vi "AK Befehl Auswerten_v1.4.vi"(10 "Array":string[](array[string])) -> (2 "String für schreiben":string)   [LabVIEW 2020, in "AK-Schnittstelle.lvlib"]
uses:
  AK-Schnittstelle.lvlib
  Aktionen Stoernummern pruefen.ctl
  Aktionen Zustandsfehlerinformation.ctl
  Aktionen Gespeicherte Werte.ctl
  Seiten/Anlagengrenzwerte/FGV Anlagengrenzwerte Aktionen.ctl
  Seiten/FT-IR/FGV FT-IR Diagnose Aktionen.ctl
  Funktionstasten/Funktionstasten-Aktion.ctl
  Seiten/System Einstellungen V2/Aktioen FGV System Konstanten.ctl
  AK Namen Aktionen.ctl
  Seiten/System Einstellungen V2/Aktioen FGV System.ctl
  Funktionstasten/Zustaende.ctl
  Seiten/Erweiterte Konfig/Status Dichtheitstest Aktionen.ctl
  Seiten/Erweiterte Konfig/FGV PID Aktionen.ctl
  Seiten/FT-IR/FGV FT-IR Aktionen.ctl
  Seiten/FT-IR/Aktion FGV Rezepte wechseln.ctl
  Seiten/FT-IR/FGV FT-IR Gasliste Aktionen.ctl
  Seiten/FT-IR/Span/Aktion FGV SGSF und SGSO weiterleiten.ctl
  Seiten/FT-IR/AK interface/Kommandos verwalten Aktionen.ctl
  Schedule Modul/Aktion FGV Scheduler Status.ctl
  PNS/Aktionen FGV Istwerte.ctl
  Funktionstasten/Betriebsart.ctl
  Seiten/FT-IR/Span/Aktion FGV Span.ctl
  Messdaten/Aktionen FGV Messdaten.ctl
  Seiten/FT-IR/AK-manuell.ctl
  Aktion FGV Spektren automatisch aufzeichnen.ctl
  Seiten/Log Konfig/Aktionen Trigger.ctl
  Seiten/Erweiterte Konfig/Dichtheitstest.vi
  Seiten/FT-IR/TOOLweb Interface Library/TOOLweb Rezept wechseln.vi
  Funktionstasten/Funktionstasten.lvlib
  Seiten/Log Konfig/LogKonfig.lvlib
  Seiten/FT-IR/FT-IR.lvlib
  Messdaten/Messdaten.lvlib
  Seiten/System Einstellungen V2/System Einstellungen V2.lvlib
  Seiten/Erweiterte Konfig/Erweiterte Konfig.lvlib
  Allgemein/allgemeine Sub-VIs.lvlib
  cRIO/PC/Kommunikation mit cRIO.lvlib
  Seiten/Anlagengrenzwerte/Anlagengrenzwerte.lvlib
  Seiten/FT-IR/TOOLweb Interface Library/TOOLweb Interface.lvlib
  PNS/PNS.lvlib
  Schedule Modul/Schedule Modul.lvlib
  Seiten/FT-IR/Span/Spanfaktor.lvlib
  Seiten/FT-IR/AK interface/AK-Interface.lvlib
  EPA 1065/Dichtheitstest 1065-345/Aktion Protokolldaten_Leak check.ctl
  EPA 1065/Dichtheitstest 1065-345/Dichtheitstest 1065-345.lvlib
  EPA 1065/Dichtheitstest 1065-345/Aktion FGV Automatic start.ctl
  Bildwechsel/Bild-Auswahl.ctl
  Bildwechsel/Bildwechsel.lvlib
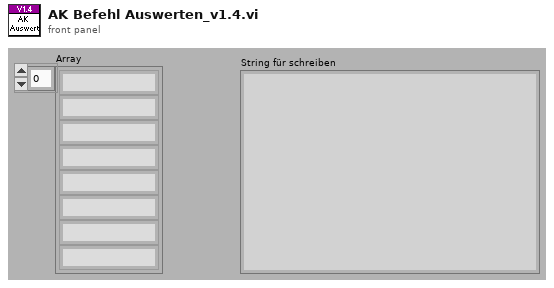
[diagram p1: front panel]
types:
  T1 = typedef "AK-Schnittstelle.lvlib/Aktionen Stoernummern pruefen.ctl" = enum16{"lesen", "prüfen"}
  T2 = typedef "AK-Schnittstelle.lvlib/Aktionen Zustandsfehlerinformation.ctl" = enum16{"OK", "Offline", "Busy", "Syntax Error", "Datenfehler"}
  T3 = typedef "AK-Schnittstelle.lvlib/Aktionen Gespeicherte Werte.ctl" = enum16{"lesen", "laden", "speichern", "Seriell", "TCP", "Diverse", "AKTIV", "AK-Namen"}
  T4 = typedef "Anlagengrenzwerte.lvlib/FGV Anlagengrenzwerte Aktionen.ctl" = enum16{"Lesen", "Grenzwerte schreiben"}
  T5 = typedef "FT-IR.lvlib/FGV FT-IR Diagnose Aktionen.ctl" = enum16{"Lesen", "Diagnose Schreiben", "Min Schreiben", "Max Schreiben"}
  T6 = typedef "Funktionstasten.lvlib/Funktionstasten-Aktion.ctl" = enum16{"Initialisieren", "Zustand setzen", "Taste gedrückt", "Fehler speichern", "Lesen", "Manuell", "Remote", "Bitparallel", "Samplepoint", "Zeit Prüfen", "reset Umschalten"}
  T7 = typedef "System Einstellungen V2.lvlib/Aktioen FGV System Konstanten.ctl" = enum16{"lesen", "laden", "speichern", "Sprache"}
  T8 = typedef "AK-Schnittstelle.lvlib/AK Namen Aktionen.ctl" = enum16{"lesen", "laden", "speichern Namen", "AK Namen", "Liste erstellen", "EKFG erstellen", "speichern EKFG", "EKFG schreiben", "Neuen Eintrag erzeugen"}
  T9 = typedef "FT-IR.lvlib/FGV FT-IR Gasliste Aktionen.ctl" = enum16{"lesen", "Gasliste FT-IR", "Gasliste ausgelesen", "laden", "speichern", "löschen"}
  T10 = typedef "System Einstellungen V2.lvlib/Aktioen FGV System.ctl" = enum16{"lesen", "laden", "speichern", "Optionen schreiben", "Zeitstempel", "Reset BMP", "Reset SQP", "Wartung", "Werkseinstellung"}
  T11 = typedef "Messdaten.lvlib/Aktionen FGV Messdaten.ctl" = enum16{"lesen", "schreiben", "löschen", "Mittelwerte", "Komponente"}
  T12 = typedef "Funktionstasten.lvlib/Zustaende.ctl" = enum16{"Standby", "Pause", "Eco", "Messen", "Kalibrieren", "Spülen Filter", "Spülen Leitung", "Umgebungsluft", "0-Gas", "Cal-Gas", "CG zu PNS", "-------------", "Init 1", "Init 2", "Init 3", "Init 4", "Messen vorbereiten", "Messen durchführen", "Exit"}
  T13 = typedef "EPA 1065.lvlib/Dichtheitstest 1065-345.lvlib/Aktion Protokolldaten_Leak check.ctl" = enum16{"lesen", "Zeitstempel", "Bearbeiter", "Daten", "Auswertung", "löschen"}
  T14 = typedef "Erweiterte Konfig.lvlib/Status Dichtheitstest Aktionen.ctl" = enum16{"lesen", "Zeitstempel", "Daten", "läuft", "Protokolldaten"}
  T15 = typedef "Erweiterte Konfig.lvlib/FGV PID Aktionen.ctl" = enum16{"Lesen", "Schreiben PID", "Schreiben Sonstige", "Dichtheitstest", "Aktionen Dicht.", "Parameter Sensor"}
  T16 = typedef "FT-IR.lvlib/FGV FT-IR Aktionen.ctl" = enum16{"lesen", "NOG setzen", "NOS setzen", "Initialisieren", "speichern", "ALLES setzen", "FT-IR Spektrum loggen", "Komm Stoppen", "Spektrum LogKonfig"}
  T17 = typedef "FT-IR.lvlib/Aktion FGV Rezepte wechseln.ctl" = enum16{"lesen", "Rezepte", "Rezeptindex", "Diesel", "Gasoline", "NCG", "laden", "speichern", "AK/Man"}
  T18 = typedef "FT-IR.lvlib/Spanfaktor.lvlib/Aktion FGV SGSF und SGSO weiterleiten.ctl" = enum16{"lesen", "AGSF", "AGSO", "AGSF löschen", "AGSO löschen", "SGSF", "SGSO", "SGSF löschen", "SGSO löschen"}
  T19 = typedef "FT-IR.lvlib/AK-Interface.lvlib/Kommandos verwalten Aktionen.ctl" = enum16{"lesen", "setzen Ende", "setzen Pos1", "senden", "initalisieren", "prüfen", "Kommandos"}
  T20 = typedef "Schedule Modul.lvlib/Aktion FGV Scheduler Status.ctl" = enum16{"lesen", "init", "aktiv", "inaktiv"}
  T21 = typedef "PNS.lvlib/Aktionen FGV Istwerte.ctl" = enum16{"lesen", "initialisieren", "schreiben", "Störungen"}
  T22 = typedef "Funktionstasten.lvlib/Betriebsart.ctl" = enum16{"Manuell", "Remote", "Bitparallel"}
  T23 = typedef "FT-IR.lvlib/Spanfaktor.lvlib/Aktion FGV Span.ctl" = enum16{"lesen", "Span", "Seite aktiv", "Offset", "FGV aktualisiert", "Aktualisierung aufheben"}
  T24 = typedef "EPA 1065.lvlib/Dichtheitstest 1065-345.lvlib/Aktion FGV Automatic start.ctl" = enum16{"lesen", "Test starten aktiv", "Test starten inaktiv", "Seite merken", "Seite zurücksetzen", "AK Start inaktiv"}
  T25 = typedef "Bildwechsel.lvlib/Bild-Auswahl.ctl" = enum16{"lesen", "Initialisieren", "Beenden", "Grafik", "Anlagenübersicht", "Anlagengrenzwerte", "Log Konfig", "Gaszuordnung AO", "Erw. Konfiguration", "FT-IR  ", "Störmeldungen", "Störmeldepuffer", "Störmeldekonfig", "PNS Grenzwerte", "Statusübersicht", "Linearisierung", "ARN", "EPA Dichtheitstest", "FID", "PMA", "CalGas", "Lambda", "Interference", "Amium PNS", "EPA T90", "Interference N2O", "Scheduler", "Systemeinstellungen", "EPA Drift"}
  T26 = typedef "FT-IR.lvlib/AK-manuell.ctl" = enum16{"manuell", "Diesel", "CNG", "Gasoline"}
  T27 = typedef "AK-Schnittstelle.lvlib/Aktion FGV Spektren automatisch aufzeichnen.ctl" = enum16{"init", "lesen", "prüfen", "set", "reset"}
  T28 = typedef "LogKonfig.lvlib/Aktionen Trigger.ctl" = enum16{"lesen", "ALLE schreiben", "Trigger prüfen", "Trigger rücksetzen"}
  T29 = typedef "AK-Schnittstelle.lvlib/Diverse gespeicherte Werte.ctl" = cluster{"Kalibriergaseingang":i16, "SamplePoint":i16, "CalGas zu PNS":i16, "Gas-Reihenfolge":i16[], "Zeit 0-Gas":sgl, "Zeit CalGas":sgl, "AK Befehlssatz":T30}
  T30 = typedef "AK-Schnittstelle.lvlib/AK Befehlssatz.ctl" = enum16{"MEXA", "IAG v1.4", "AVL (Puma)", "PEUS"}
  T31 = typedef "Anlagengrenzwerte.lvlib/Anlagen-Grenzwerte Anzeige.ctl" = cluster{"Eingangsdruck FT-IR:":T32, "Durchfluss FT-IR:":T32, "Durchfluss CalGas:":T32, "Druck Ausgang:":T32, "Druck Kalter Block:":T32, "Heizleitungen intern:":T32, "Heizleitung zu FT-IR:":T32, "Heizung Filterblock:":T32, "Heizung Pumpe:":T32, "Heizleitung Extern SP1:":T32, "Heizleitung Extern SP2:":T32, "FT-IR Heizung Messzelle:":T32, "Schaltschranktemperatur:":T32, "Gaskühler:":T32}
  T32 = typedef "Anlagengrenzwerte.lvlib/Anlagen-Parameter Anzeige.ctl" = cluster{"Sollwert":sgl, "Warn-Min":sgl, "Warn-Max":sgl, "Abschalt-Min":sgl, "Abschalt-Max":sgl, "Regler":u16}
  T33 = typedef "Verwaltung - cRIO.lvlib/Analog Eingaenge.ctl" = cluster{"AI0: Durchfluss FT-IR":sgl, "AI1: Druck Ausgang":sgl, "AI2: Umgebungsdruck":sgl, "AI3: Druck FT-IR":sgl, "AI4: Druck CalGas":sgl, "AI5: Reserve":sgl, "AI6: Reserve":sgl, "AI7: Reserve":sgl, "Rohwert Durchfluss FT-IR":sgl, "Rohwert Druck Ausgang":sgl, "Rohwert Umgebungsdruck":sgl, "Rohwert Druck FT-IR":sgl, "Rohwert Druck CalGas":sgl, "Rohwert AI5":sgl, "Rohwert AI6":sgl, "Rohwert AI7":sgl, "Rohwert Diffdruck mbar FTIR":sgl}
  T34 = typedef "FT-IR.lvlib/TOOLweb Interface.lvlib/Typdefinitionen.lvlib/TOOLweb Diagnose.ctl" = cluster{"(14) temperature":sgl, "(15) pressure":sgl, "(16) oxygen":sgl, "(50) diag-igramdc":sgl, "(51) diag-igrampp":sgl, "(52) diag-phaseAngle":sgl, "(53) diag-laserpp":sgl, "(54) diag-laserdc":sgl, "(55) diag-badscan":sgl, "(56) diag-centerburst":sgl, "(57) diag-linearizerCheck":sgl, "(58) diag-SNR":sgl, "(59) diag-sBeamIntensity":sgl}
  T35 = cluster{"Modell":string, "ProjektNummer":string, "Software Version":string, "Seriennummer":string}
  T36 = typedef "String - Ausgabefeld.ctl" = string
  T37 = typedef "System Einstellungen V2.lvlib/Optionen.ctl" = cluster{"Störmeldep.":bool, "Betriebszustände":bool, "AK in ppm":bool, "log Cal-Gas":bool, "log 0-Gas":bool, "Durchflusssensor 0-5V":bool, "PNS?":bool, "Mit N2 spülen":bool, "TRE08":bool, "Amium 10-Fach":bool, "Verticale Scrollbar aktiv":bool, "Loggingtakt":bool, "AK Rezeptwechsel gleich wie MKS":bool, "NG ECO":bool}
  T38 = typedef "EPA 1065.lvlib/Dichtheitstest 1065-345.lvlib/Leak Daten.ctl" = cluster{"Gesamtes Volumen":sgl, "p 1":sgl, "p 2":sgl, "T 1":sgl, "T 2":sgl, "t 1":timestamp, "t 2":timestamp, "Ergebnis mol/s":sgl, "Grenze mol/s":sgl, "Leak in %":sgl, "Ergebnis mbar":sgl, "Grenze mbar":sgl}
  T39 = typedef "Erweiterte Konfig.lvlib/Sonstige Parameter.ctl" = cluster{"Lüfter langsam":sgl, "Lüfter schnell":sgl, "FT-IR Kühlung Soll":sgl, "FT-IR Kühlung Max":sgl, "Überwachung":T40, "Befüllung aktiv":T41, "Stickstoff Befüllzeit":sgl, "Befüllintervall":sgl, "Kalibrierwert FT-IR":sgl, "Offset Ausgang":sgl, "Offset FT-IR":sgl, "Offset Druck FT-IR":sgl, "Dichtheitstest Zeit":sgl, "Dichtheitstest Abfall":sgl, "Dichtheitstest Umfang":T42, "Offset Umgebung":sgl, "Max Taupunkt":sgl, "Pumpendrehzahl":sgl, "ext. Befüllung":T41, "Ext. Stickstoff Befüllzeit":sgl}
  T40 = typedef "Auswahlfeld.ctl" = u16
  T41 = typedef "LogKonfig.lvlib/Auswahlfeld aktiviert-deaktiviert.ctl" = u16
  T42 = typedef "Erweiterte Konfig.lvlib/Dichtheitstest Umfang.ctl" = u16
  T43 = cluster{"(80) labEnabled":bool, "(81) labPath":path, "(82) labBaseName":string, "(83) labIndex":string, "Spektrum loggen aktiv?":bool}
  T44 = typedef "Verwaltung - cRIO.lvlib/TC Eingaenge.ctl" = cluster{"TC0: Reserve":sgl, "TC1: HL zu FT-IR":sgl, "TC2: HL Extern SP1":sgl, "TC3: HL Extern SP2":sgl, "TC4: Reserve":sgl, "TC5: Reserve":sgl, "TC6: Reserve":sgl, "TC7: Reserve":sgl, "TC8: FT-IR":sgl, "TC9: Reserve":sgl, "TC10: Schaltschrank":sgl, "TC11: Umgebung":sgl}
  T45 = typedef "Steuerung PNS.lvclass/Regler.ctl" = cluster{"Istwert":i16, "Sollwert":i16, "Alarm MIN":i16, "Alarm MAX":i16, "Regler sperren":i16, "Analog Ausgang":i16}[]
  T46 = cluster{"Istwert":i16, "Sollwert":i16, "Alarm MIN":i16, "Alarm MAX":i16, "Regler sperren":i16, "Analog Ausgang":i16}
  T47 = typedef "LogKonfig.lvlib/Element Triggerereignisse.ctl" = cluster{"Trigger verwenden":T41, "Messwert":u16, "kl./gr.":u16, "Wert":sgl, "Puffergröße":sgl}
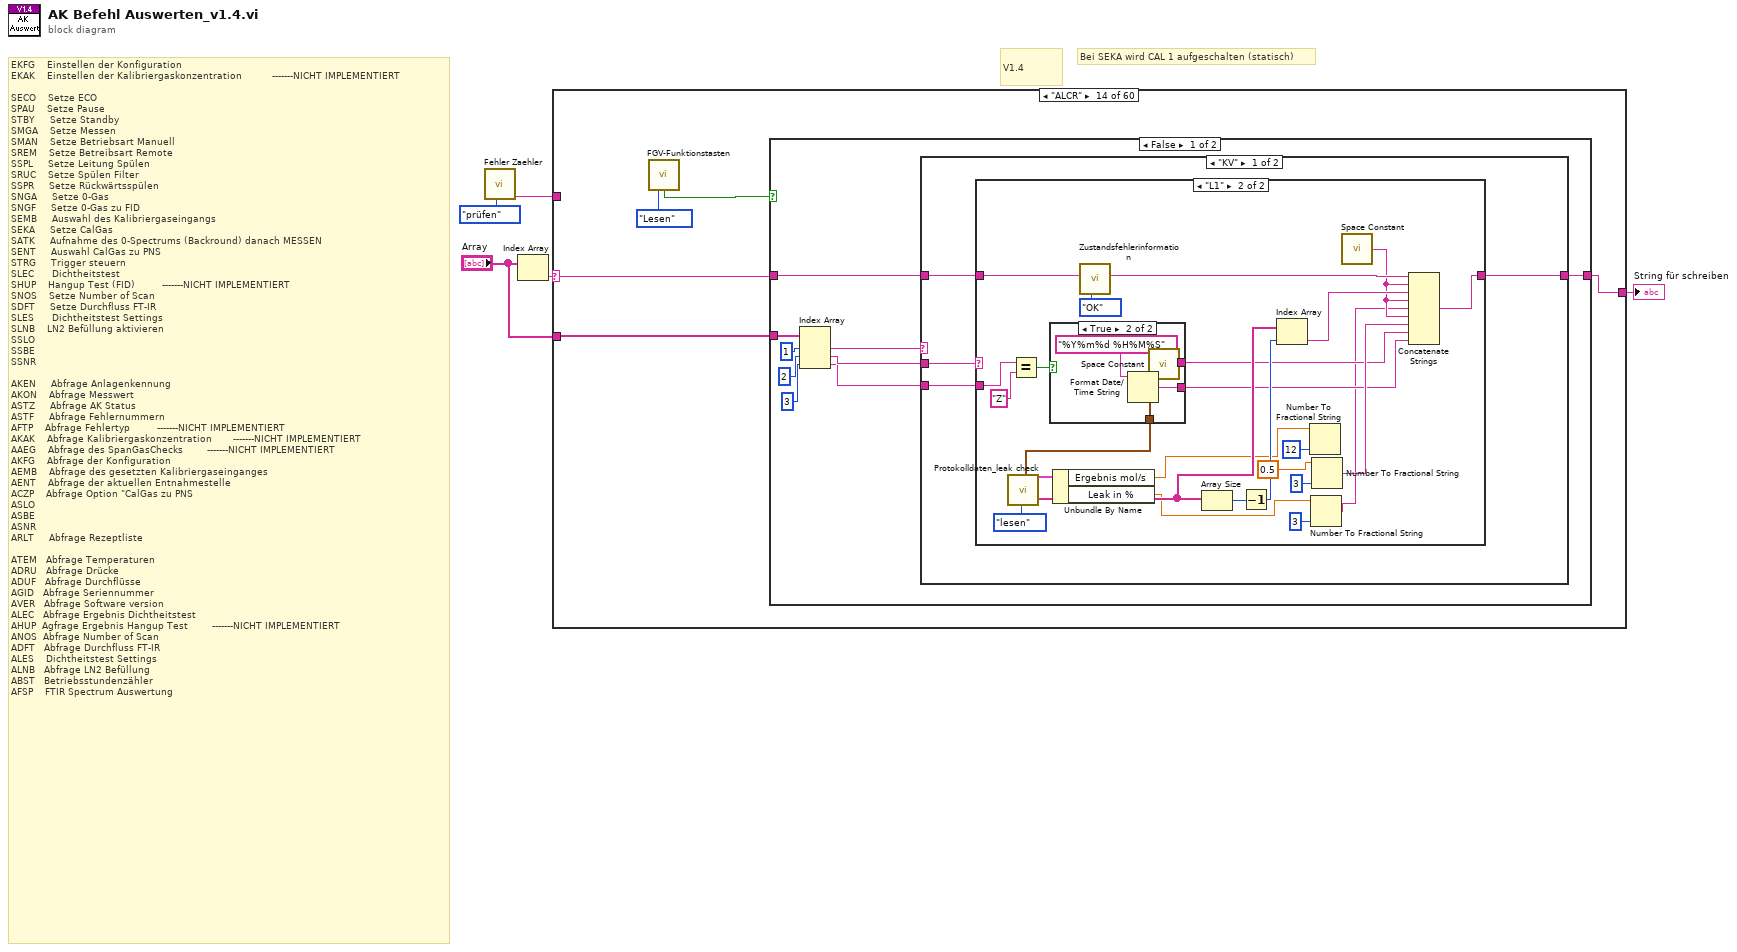
[diagram p0: block diagram]
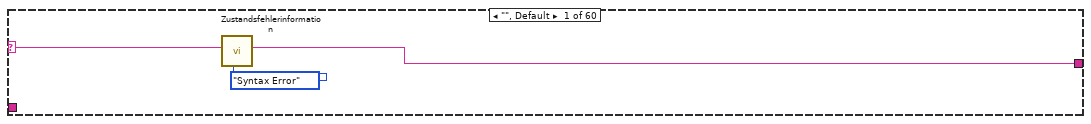
[diagram p2: hidden frame]
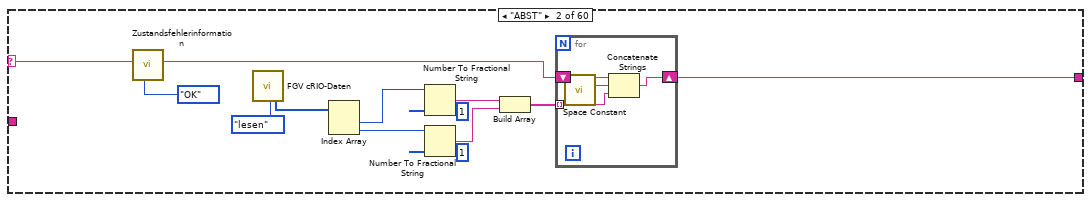
[diagram p3: hidden frame]
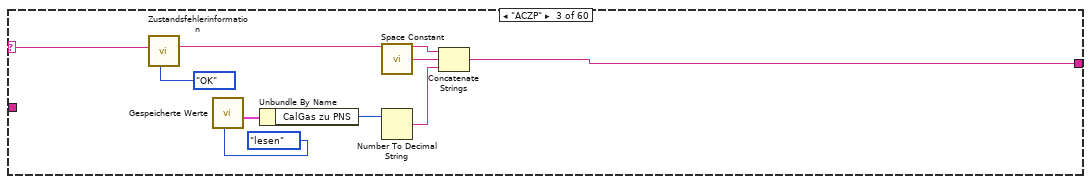
[diagram p4: hidden frame]
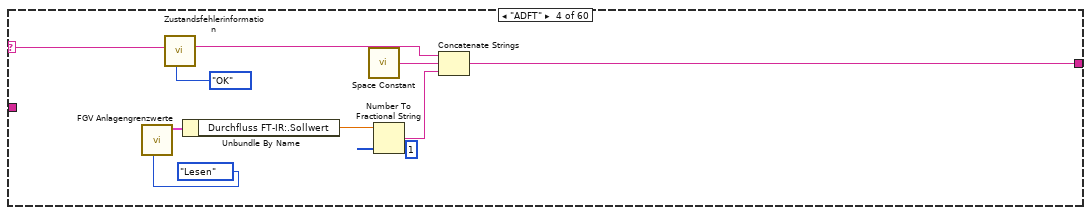
[diagram p5: hidden frame]
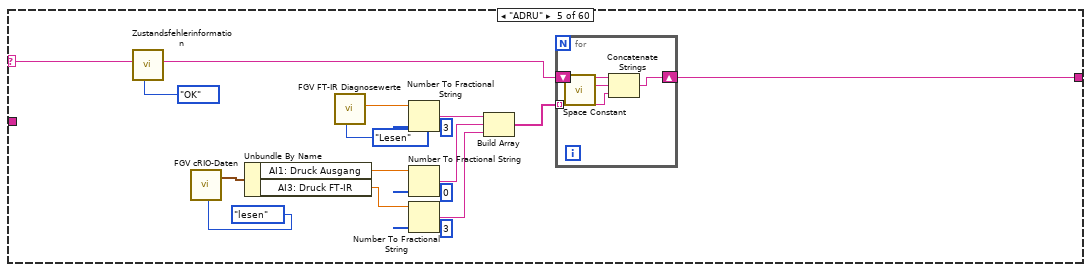
[diagram p6: hidden frame]
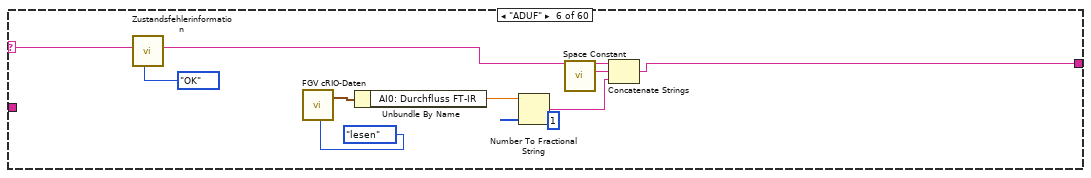
[diagram p7: hidden frame]
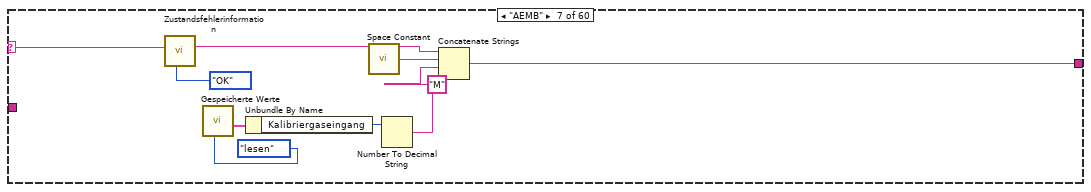
[diagram p8: hidden frame]
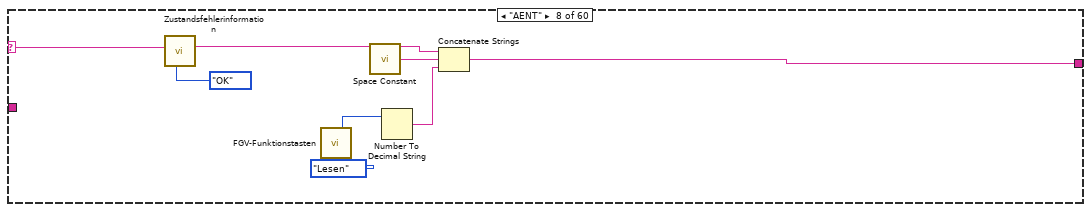
[diagram p9: hidden frame]
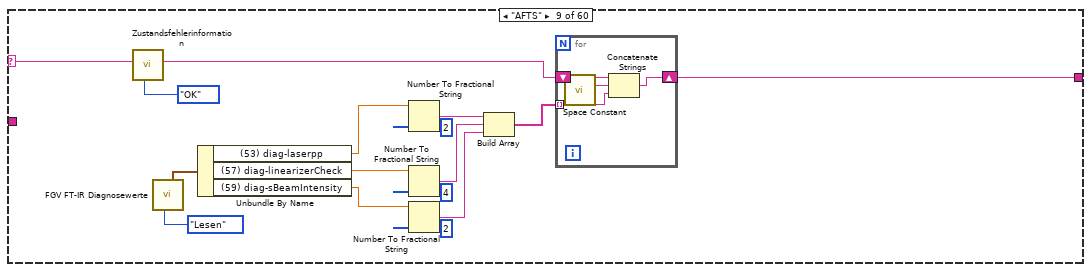
[diagram p10: hidden frame]
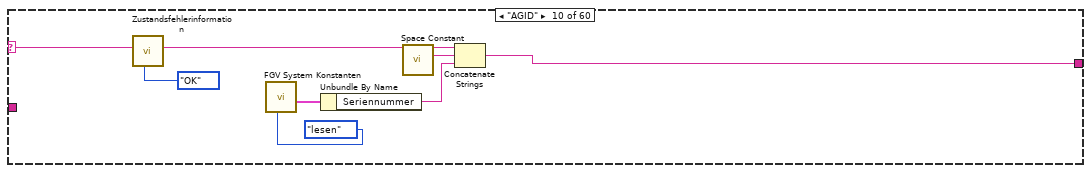
[diagram p11: hidden frame]
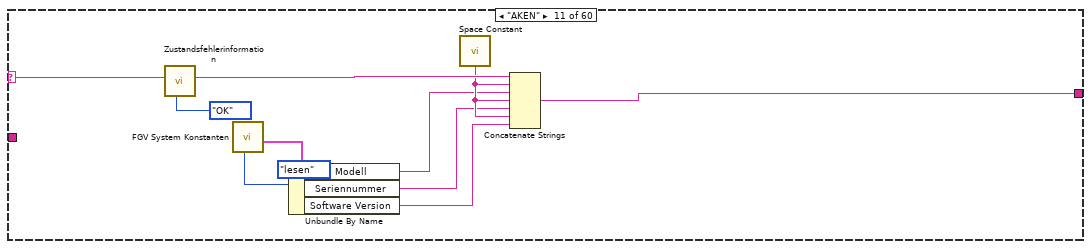
[diagram p12: hidden frame]
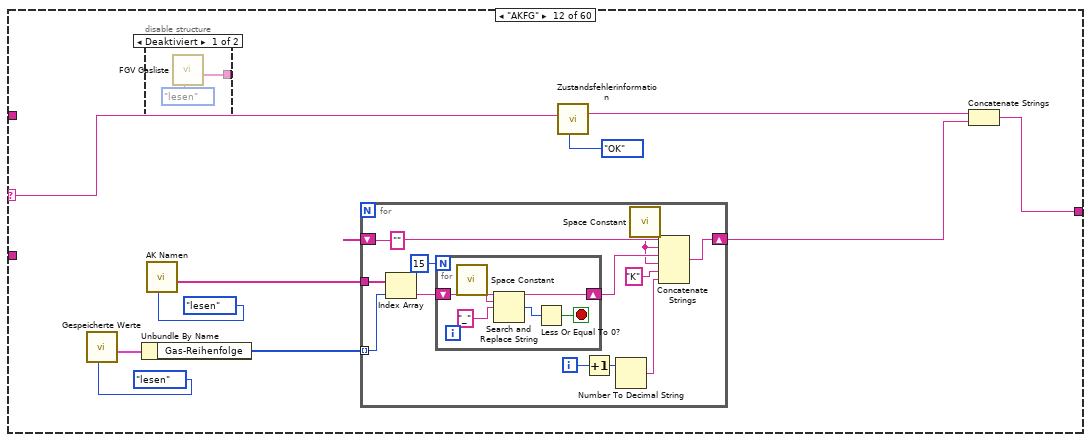
[diagram p13: hidden frame]
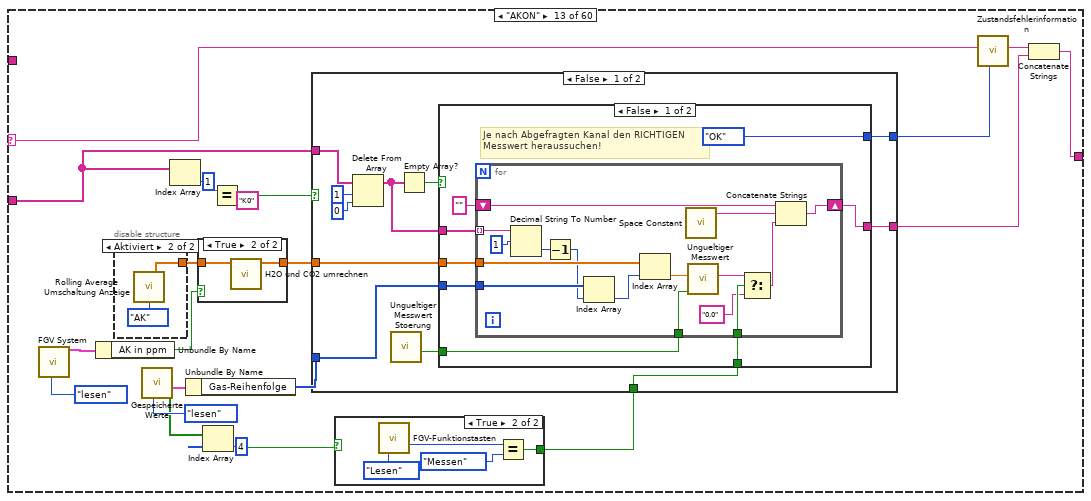
[diagram p15: hidden frame]
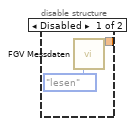
[diagram p16: hidden frame]
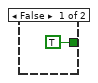
[diagram p17: hidden frame]
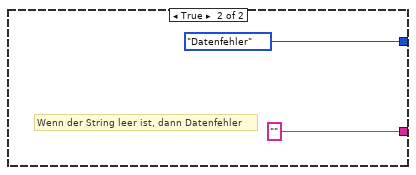
[diagram p19: hidden frame]
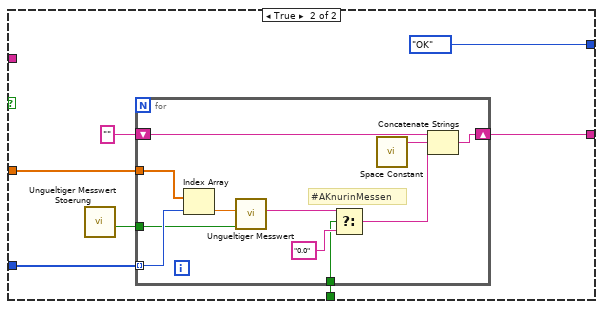
[diagram p20: hidden frame]
diagram:
  # "Bei SEKA wird CAL 1 aufgeschalten (statisch)"
  # "V1.4"
  # "EKFG    Einstellen der Konfiguration\nEKAK    Einstellen der Kalibriergaskonzentration          -------NICHT IMPLEMENTIERT\n\nSECO    Setze ECO\nSPAU    Setze Pause\nSTBY     Setze Standby\nSMGA    Setze Messen\nSMAN    Setze Betriebsart Manuell\nSREM    Setze Betreibsart Remote\nSSPL     Setze Leitung Spülen\nSRUC    Setze Spülen Filter\nSSPR     Setze Rückwärtsspülen\nSNGA     Setze 0-Gas\nSNGF     Setze 0-Gas zu FID\nSEMB     Auswahl des Kalibriergaseingangs\nSEKA     Setze CalGas\nSATK     Aufnahme des 0-Spectrums (Backround) danach MESSEN\nSENT     Auswahl CalGas zu PNS\nSTRG     Trigger steuern\nSLEC      Dichtheitstest\nSHUP    Hangup Test (FID)         -------NICHT IMPLEMENTIERT\nSNOS    Setze Number of Scan\nSDFT     Setze Durchfluss FT-IR\nSLES      Dichtheitstest Settings\nSLNB    LN2 Befüllung aktivieren\nSSLO\nSSBE\nSSNR\n\nAKEN     Abfrage Anlagenkennung\nAKON    Abfrage Messwert\nASTZ     Abfrage AK Status\nASTF     Abfrage Fehlernummern\nAFTP    Abfrage Fehlertyp         -------NICHT IMPLEMENTIERT\nAKAK    Abfrage Kalibriergaskonzentration       -------NICHT IMPLEMENTIERT\nAAEG    Abfrage des SpanGasChecks        -------NICHT IMPLEMENTIERT\nAKFG    Abfrage der Konfiguration\nAEMB    Abfrage des gesetzten Kalibriergaseinganges\nAENT    Abfrage der aktuellen Entnahmestelle\nACZP    Abfrage Option \"CalGas zu PNS\nASLO\nASBE\nASNR\nARLT     Abfrage Rezeptliste\n\nATEM   Abfrage Temperaturen\nADRU   Abfrage Drücke\nADUF   Abfrage Durchflüsse\nAGID   Abfrage Seriennummer\nAVER   Abfrage Software version\nALEC   Abfrage Ergebnis Dichtheitstest\nAHUP  Agfrage Ergebnis Hangup Test        -------NICHT IMPLEMENTIERT\nANOS  Abfrage Number of Scan\nADFT   Abfrage Durchfluss FT-IR\nALES    Dichtheitstest Settings\nALNB   Abfrage LN2 Befüllung\nABST   Betriebsstundenzähler\nAFSP    FTIR Spectrum Auswertung"
  n1 = call "Fehler Zaehler.vi"("Aktionen"=Aktionen_Stoernummern_pruefen."prüfen") -> ("Fehlerzähler"=w3:string)  [unwired: 7 in, 3 out]
  n2 = Index Array(array="Array") -> (element=w2:string)  [unwired: 1 in]
  n3 = case shown="\"ALCR\"" w2 {
    selector: w2 -> [w7 w20 w32 w42 w60 w74 w83 w91 w108 w120 w129 w140 w183 w252 w321 w342 w354 w362 w369 w386 w410 w420 w453 w486 w519 w548 w558 w566 w573 w585 w627 w642 w650 w668 w673 w701 w858 w860 w891 w913 w933 w970 w994 w1045 w1075 w1089 w1099 w1103 w1106 w1137 w1144 w1216 w1228 w1235 w1270 w1320 w1352 w1356 w1359 w1362]
    tunnel: [w6 w18 w34 w44 w55 w71 w85 w93 w106 w116 w131 w142 w184 w253 w314 w340 w356 w364 w371 w373 w399 w416 w449 w482 w515 w550 w560 w568 w575 w587 w620 w638 w649 w667 w672 w700 w857 w859 w890 w912 w934 w969 w993 w1044 w1074 w1088 w1098 w1102 w1105 w1136 w1143 w1215 w1227 w1234 w1269 w1319 w1351 w1355 w1358 w1361] -> w5
    tunnel: w3 -> [_ _ _ _ _ _ _ _ _ _ _ _ _ _ _ _ _ _ _ _ _ _ _ _ _ _ _ _ _ _ _ _ _ _ _ _ _ _ _ _ _ _ _ _ _ _ _ _ _ _ _ _ _ _ _ _ _ _ _ _]
    tunnel: "Array" -> [_ _ _ _ _ _ _ _ _ _ _ _ w174 w254 _ _ _ _ _ _ _ w425 w458 w491 w524 _ _ _ _ _ _ _ w651 _ w671 w705 _ _ w889 w911 w935 _ w992 w1043 _ _ w1097 _ w1104 _ w1145 _ w1220 w1230 w1265 w1315 w1344 _ _ w1360]
    frame "", Default {
      n4 = call "Zustandsfehlerinformation.vi"("Aktionen"=Aktionen_Zustandsfehlerinformation."Syntax Error", "String"=w7) -> ("String"=w6:string)  [unwired: 9 in]
    }
    frame "ABST" {
      n5 = call "Zustandsfehlerinformation.vi"("Aktionen"=Aktionen_Zustandsfehlerinformation."OK", "String"=w20) -> ("String"=w17:string)  [unwired: 9 in]
      n6 = call "FGV cRIO-Daten.vi"("Aktion"=enum16{"lesen", "schreiben"}."lesen") -> ("PID Stellwerte"=w9:i16[])  [unwired: 9 in, 9 out]
      n7 = Index Array(array=w9) -> (element #1=w10:i16, element #2=w11:i16)  [unwired: 2 in]
      n8 = Number To Fractional String(number=w10, precision (6)=i16 1 ("Genauigkeit (6)")) -> (F-format string=w14:string)  [unwired: 2 in]
      n9 = Number To Fractional String(number=w11, precision (6)=i16 1 ("Genauigkeit (6)")) -> (F-format string=w13:string)  [unwired: 2 in]
      n10 = Build Array(w14, w13) -> (w19:string[])
      n11 = for {
        tunnel: w19 -> [w22] mode=indexing
        shift-right: [w23] -> w18
        shift-left: w17 -> [w25]
        n12 = call <vilib>:"Space Constant.vi"() -> ("String"=w24:string)
        n13 = Concatenate Strings(w25, w24, w22) -> (w23:string)
      }
    }
    frame "ACZP" {
      n14 = call "Zustandsfehlerinformation.vi"("Aktionen"=Aktionen_Zustandsfehlerinformation."OK", "String"=w32) -> ("String"=w31:string)  [unwired: 9 in]
      n15 = call "Gespeicherte Werte.vi"("Aktionen"=Aktionen_Gespeicherte_Werte."lesen") -> ("Diverse Werte"=w26:T29)  [unwired: 6 in, 4 out]
      n16 = Unbundle By Name(w26) -> ("CalGas zu PNS"=w29:i16)
      n17 = call <vilib>:"Space Constant.vi"() -> ("String"=w27:string)
      n18 = Number To Decimal String(number=w29) -> (decimal integer string=w28:string)  [unwired: 1 in]
      n19 = Concatenate Strings(w31, w27, w28) -> (w34:string)
    }
    frame "ADFT" {
      n20 = call "FGV Anlagengrenzwerte.vi"("Aktion"=FGV_Anlagengrenzwerte_Aktionen."Lesen") -> ("Anlagen-Grenzwerte Anzeige"=w38:T31)  [unwired: 1 in, 9 out]
      n21 = call "Zustandsfehlerinformation.vi"("Aktionen"=Aktionen_Zustandsfehlerinformation."OK", "String"=w42) -> ("String"=w41:string)  [unwired: 9 in]
      n22 = Unbundle By Name(w38) -> ("Durchfluss FT-IR:.Sollwert"=w37:sgl)
      n23 = call <vilib>:"Space Constant.vi"() -> ("String"=w40:string)
      n24 = Number To Fractional String(number=w37, precision (6)=i16 1 ("Genauigkeit (6)")) -> (F-format string=w35:string)  [unwired: 2 in]
      n25 = Concatenate Strings(w41, w40, w35) -> (w44:string)
    }
    frame "ADRU" {
      n26 = call "Zustandsfehlerinformation.vi"("Aktionen"=Aktionen_Zustandsfehlerinformation."OK", "String"=w60) -> ("String"=w54:string)  [unwired: 9 in]
      n27 = call "FGV cRIO-Daten.vi"("Aktion"=enum16{"lesen", "schreiben"}."lesen") -> ("Analog Input"=w58:T33)  [unwired: 9 in, 9 out]
      n28 = Unbundle By Name(w58) -> ("AI1: Druck Ausgang"=w50:sgl, "AI3: Druck FT-IR"=w48:sgl)
      n29 = call "FGV FT-IR Diagnosewerte.vi"("Aktionen"=FGV_FT-IR_Diagnose_Aktionen."Lesen") -> ("Druck"=w52:dbl)  [unwired: 5 in, 5 out]
      n30 = Number To Fractional String(number=w52, precision (6)=i16 3 ("Genauigkeit (6)")) -> (F-format string=w47:string)  [unwired: 2 in]
      n31 = Number To Fractional String(number=w50, precision (6)=i16 0 ("Genauigkeit (6)")) -> (F-format string=w45:string)  [unwired: 2 in]
      n32 = Number To Fractional String(number=w48, precision (6)=i16 3 ("Genauigkeit (6)")) -> (F-format string=w46:string)  [unwired: 2 in]
      n33 = Build Array(w47, w45, w46) -> (w56:string[])
      n34 = for {
        tunnel: w56 -> [w62] mode=indexing
        shift-right: [w63] -> w55
        shift-left: w54 -> [w65]
        n35 = call <vilib>:"Space Constant.vi"() -> ("String"=w64:string)
        n36 = Concatenate Strings(w65, w64, w62) -> (w63:string)
      }
    }
    frame "ADUF" {
      n37 = call "Zustandsfehlerinformation.vi"("Aktionen"=Aktionen_Zustandsfehlerinformation."OK", "String"=w74) -> ("String"=w70:string)  [unwired: 9 in]
      n38 = call "FGV cRIO-Daten.vi"("Aktion"=enum16{"lesen", "schreiben"}."lesen") -> ("Analog Input"=w73:T33)  [unwired: 9 in, 9 out]
      n39 = Unbundle By Name(w73) -> ("AI0: Durchfluss FT-IR"=w69:sgl)
      n40 = Number To Fractional String(number=w69, precision (6)=i16 1 ("Genauigkeit (6)")) -> (F-format string=w66:string)  [unwired: 2 in]
      n41 = call <vilib>:"Space Constant.vi"() -> ("String"=w67:string)
      n42 = Concatenate Strings(w70, w67, w66) -> (w71:string)
    }
    frame "AEMB" {
      n43 = call "Zustandsfehlerinformation.vi"("Aktionen"=Aktionen_Zustandsfehlerinformation."OK", "String"=w83) -> ("String"=w82:string)  [unwired: 9 in]
      n44 = call "Gespeicherte Werte.vi"("Aktionen"=Aktionen_Gespeicherte_Werte."lesen") -> ("Diverse Werte"=w76:T29)  [unwired: 6 in, 4 out]
      n45 = Unbundle By Name(w76) -> ("Kalibriergaseingang"=w80:i16)
      n46 = call <vilib>:"Space Constant.vi"() -> ("String"=w77:string)
      n47 = Number To Decimal String(number=w80) -> (decimal integer string=w78:string)  [unwired: 1 in]
      n48 = Concatenate Strings(w82, w77, "M" ("String"), w78) -> (w85:string)
    }
    frame "AENT" {
      n49 = call "Zustandsfehlerinformation.vi"("Aktionen"=Aktionen_Zustandsfehlerinformation."OK", "String"=w91) -> ("String"=w90:string)  [unwired: 9 in]
      n50 = call "FGV-Funktionstasten.vi"("Aktion"=Funktionstasten-Aktion."Lesen") -> ("Samplepoint"=w86:u16)  [unwired: 7 in, 7 out]
      n51 = call <vilib>:"Space Constant.vi"() -> ("String"=w88:string)
      n52 = Number To Decimal String(number=w86) -> (decimal integer string=w89:string)  [unwired: 1 in]
      n53 = Concatenate Strings(w90, w88, w89) -> (w93:string)
    }
    frame "AFTS" {
      n54 = call "Zustandsfehlerinformation.vi"("Aktionen"=Aktionen_Zustandsfehlerinformation."OK", "String"=w108) -> ("String"=w105:string)  [unwired: 9 in]
      n55 = call "FGV FT-IR Diagnosewerte.vi"("Aktionen"=FGV_FT-IR_Diagnose_Aktionen."Lesen") -> ("Diagnose"=w98:T34)  [unwired: 5 in, 5 out]
      n56 = Unbundle By Name(w98) -> ("(53) diag-laserpp"=w96:sgl, "(57) diag-linearizerCheck"=w95:sgl, "(59) diag-sBeamIntensity"=w94:sgl)
      n57 = Number To Fractional String(number=w96, precision (6)=i16 2 ("Genauigkeit (6)")) -> (F-format string=w101:string)  [unwired: 2 in]
      n58 = Number To Fractional String(number=w95, precision (6)=i16 4 ("Genauigkeit (6)")) -> (F-format string=w99:string)  [unwired: 2 in]
      n59 = Number To Fractional String(number=w94, precision (6)=i16 2 ("Genauigkeit (6)")) -> (F-format string=w100:string)  [unwired: 2 in]
      n60 = Build Array(w101, w99, w100) -> (w107:string[])
      n61 = for {
        tunnel: w107 -> [w110] mode=indexing
        shift-right: [w111] -> w106
        shift-left: w105 -> [w113]
        n62 = call <vilib>:"Space Constant.vi"() -> ("String"=w112:string)
        n63 = Concatenate Strings(w113, w112, w110) -> (w111:string)
      }
    }
    frame "AGID" {
      n64 = call "Zustandsfehlerinformation.vi"("Aktionen"=Aktionen_Zustandsfehlerinformation."OK", "String"=w120) -> ("String"=w117:string)  [unwired: 9 in]
      n65 = call "FGV System Konstanten.vi"("Aktionen"=Aktioen_FGV_System_Konstanten."lesen") -> ("Cluster out"=w115:T35)  [unwired: 6 in, 4 out]
      n66 = Unbundle By Name(w115) -> ("Seriennummer"=w114:string)
      n67 = call <vilib>:"Space Constant.vi"() -> ("String"=w119:string)
      n68 = Concatenate Strings(w117, w119, w114) -> (w116:string)
    }
    frame "AKEN" {
      n69 = call "Zustandsfehlerinformation.vi"("Aktionen"=Aktionen_Zustandsfehlerinformation."OK", "String"=w129) -> ("String"=w128:string)  [unwired: 9 in]
      n70 = call "FGV System Konstanten.vi"("Aktionen"=Aktioen_FGV_System_Konstanten."lesen") -> ("Cluster out"=w125:T35)  [unwired: 6 in, 4 out]
      n71 = Unbundle By Name(w125) -> ("Modell"=w122:string, "Seriennummer"=w124:string, "Software Version"=w123:string)
      n72 = call <vilib>:"Space Constant.vi"() -> ("String"=w126:string)
      n73 = Concatenate Strings(w128, w126, w122, w126, w124, w126, w123) -> (w131:string)
    }
    frame "AKFG" {
      n74 = call "Gespeicherte Werte.vi"("Aktionen"=Aktionen_Gespeicherte_Werte."lesen") -> ("Diverse Werte"=w136:T29)  [unwired: 6 in, 4 out]
      n75 = Unbundle By Name(w136) -> ("Gas-Reihenfolge"=w138:i16[])
      n76 = disable-structure shown="Deaktiviert" {
        disable-tunnel: [w161 _] -> _
        frame Disabled {
          n77 = call "FGV Gasliste.vi"("Aktionen"=FGV_FT-IR_Gasliste_Aktionen."lesen") -> ("Aktuelle Gasliste gesamt"=w161:T36[])  [unwired: 8 in, 2 out]
        }
        frame Enabled {
        }
      }
      n78 = call "AK Namen.vi"("Aktionen"=AK_Namen_Aktionen."lesen") -> ("AK Namen"=w132:string[])  [unwired: 7 in, 3 out]
      n79 = for {
        tunnel: w138 -> [w151] mode=indexing
        shift-right: [w154] -> w135
        shift-left: "" -> [w153]
        tunnel: w132 -> [w152]
        i -> [w145]
        n80 = Index Array(array=w152, index=w151) -> (element=w149:string)
        n81 = for {
          N: 15 -> [_]
          shift-right: [w159] -> w148
          shift-left: w149 -> [w160]
          stop <- w157 stop-if-true
          n82 = call <vilib>:"Space Constant.vi"() -> ("String"=w156:string)
          n83 = Search and Replace String(input string=w160, search string=w156, replace string="_") -> (result string=w159:string, number of replacements=w158:i32)  [unwired: 5 in, 2 out]
          n84 = Less Or Equal To 0?(x=w158) -> (x <= 0?=w157:bool)
        }
        n85 = Increment(x=w145) -> (x+1=w144:i32)
        n86 = Number To Decimal String(number=w144) -> (decimal integer string=w143:string)  [unwired: 1 in]
        n87 = call <vilib>:"Space Constant.vi"() -> ("String"=w147:string)
        n88 = Concatenate Strings(w153, w147, w148, w147, "K" ("String"), w143) -> (w154:string)
      }
      n89 = call "Zustandsfehlerinformation.vi"("Aktionen"=Aktionen_Zustandsfehlerinformation."OK", "String"=w140) -> ("String"=w139:string)  [unwired: 9 in]
      n90 = Concatenate Strings(w139, w135) -> (w142:string)
    }
    frame "AKON" {
      n91 = call "FGV System.vi"("Aktionen"=Aktioen_FGV_System."lesen") -> ("Optionen"=w168:T37)  [unwired: 12 in, 6 out]
      n92 = Unbundle By Name(w168) -> ("AK in ppm"=w171:bool)
      n93 = disable-structure shown="Aktiviert" {
        disable-tunnel: [w186 w188] -> w170
        frame Disabled {
          n94 = call "FGV Messdaten.vi"("Aktionen"=Aktionen_FGV_Messdaten."lesen") -> ("Aktuelle Messwerte"=w186:sgl[])  [unwired: 6 in, 8 out]
        }
        frame Enabled {
          n95 = call "Rolling Average Umschaltung Anzeige.vi"("Aktion"=enum16{"AK", "IAG Software"}."AK") -> ("Aktuelle Messwerte"=w188:sgl[])  [unwired: 9 in, 5 out]
        }
      }
      n96 = call "Gespeicherte Werte.vi"("Aktionen"=Aktionen_Gespeicherte_Werte."lesen") -> ("AKTIV?"=w165:bool[], "Diverse Werte"=w172:T29)  [unwired: 6 in, 3 out]
      n97 = Index Array(array=w174, index=1 ("Index")) -> (element=w177:string)
      n98 = Unbundle By Name(w172) -> ("Gas-Reihenfolge"=w180:i16[])
      n99 = case shown="True" w171 {
        tunnel: w170 -> [w194 w196]
        tunnel: [w194 w195] -> w167
        frame False {
        }
        frame True {
          n100 = call "H2O und CO2 umrechnen.vi"("Aktuelle Messwerte"=w196) -> ("Aktuelle Messwerte"=w195:sgl[])  [unwired: 10 in]
        }
      }
      n101 = Index Array(array=w165, index=4 ("Index")) -> (element=w163:bool)
      n102 = Equal?(x=w177, y="K0") -> (x = y?=w175:bool)
      n103 = case shown="True" w163 {
        tunnel: [TRUE w190] -> w166
        frame False {
        }
        frame True {
          n104 = call "FGV-Funktionstasten.vi"("Aktion"=Funktionstasten-Aktion."Lesen") -> ("ausgewählte Funktion"=w192:T12)  [unwired: 7 in, 7 out]
          n105 = Equal?(x=w192, y=Zustaende."Messen") -> (x = y?=w190:bool)
        }
      }
      n106 = case shown="False" w175 {
        tunnel: w180 -> [w201 w240]
        tunnel: [w199 w238] -> w179
        tunnel: w167 -> [w200 w237]
        tunnel: w174 -> [w205 _]
        tunnel: [w203 Aktionen_Zustandsfehlerinformation."OK" ("Aktionen")] -> w173
        tunnel: w166 -> [w197 w234]
        frame False {
          n107 = Delete From Array(array=w205, length=1 ("Länge"), index=0 ("Index")) -> (array with subset deleted=w202:string[])  [unwired: 1 out]
          n108 = call "Ungueltiger Messwert Stoerung.vi"() -> ("Störung Messgerät"=w198:bool)  [unwired: 11 in]
          n109 = Empty Array?(array=w202) -> (empty?=w204:bool)
          n110 = case shown="False" w204 {
            tunnel: [Aktionen_Zustandsfehlerinformation."OK" ("Aktionen") Aktionen_Zustandsfehlerinformation."Datenfehler" ("Aktionen")] -> w203
            tunnel: w202 -> [w214 _]
            tunnel: w201 -> [w213 _]
            tunnel: w200 -> [w212 _]
            tunnel: [w211 ""] -> w199
            tunnel: w198 -> [w209 _]
            tunnel: w197 -> [w208 _]
            frame False {
              # "Je nach Abgefragten Kanal den RICHTIGEN\nMesswert heraussuchen!"
              n111 = for {
                tunnel: w214 -> [w231] mode=indexing
                tunnel: w213 -> [w229]
                tunnel: w212 -> [w228]
                shift-right: [w227] -> w211
                shift-left: "" -> [w226]
                tunnel: w209 -> [w220]
                tunnel: w208 -> [w218]
                n112 = Decimal String To Number(string=w231, offset=1 ("Offset (0)")) -> (number=w225:i32)  [unwired: 1 in, 1 out]
                n113 = Decrement(x=w225) -> (x-1=w224:i32)
                n114 = Index Array(array=w229, index=w224) -> (element=w222:i16)
                n115 = Index Array(array=w228, index=w222) -> (element=w221:sgl)
                n116 = call <vilib>:"Space Constant.vi"() -> ("String"=w223:string)
                n117 = call "Ungueltiger Messwert.vi"("Stöung Messgerät"=w220, "Messwert"=w221) -> ("Messwert String"=w217:string)  [unwired: 9 in]
                n118 = Select(t=w217, s=w218, f="0.0") -> (s? t:f=w219:string)
                n119 = Concatenate Strings(w226, w223, w219) -> (w227:string)
              }
            }
            frame True {
              # "Wenn der String leer ist, dann Datenfehler"
            }
          }
        }
        frame True {
          n120 = call "Ungueltiger Messwert Stoerung.vi"() -> ("Störung Messgerät"=w235:bool)  [unwired: 11 in]
          n121 = for {
            tunnel: w240 -> [w247] mode=indexing
            shift-right: [w251] -> w238
            shift-left: "" -> [w250]
            tunnel: w237 -> [w249]
            tunnel: w235 -> [w245]
            tunnel: w234 -> [w243]
            # "#AKnurinMessen"
            n122 = Index Array(array=w249, index=w247) -> (element=w246:sgl)
            n123 = call "Ungueltiger Messwert.vi"("Stöung Messgerät"=w245, "Messwert"=w246) -> ("Messwert String"=w242:string)  [unwired: 9 in]
            n124 = Select(t=w242, s=w243, f="0.0") -> (s? t:f=w241:string)
            n125 = call <vilib>:"Space Constant.vi"() -> ("String"=w248:string)
            n126 = Concatenate Strings(w250, w248, w241) -> (w251:string)
          }
        }
      }
      n127 = call "Zustandsfehlerinformation.vi"("Aktionen"=w173, "String"=w183) -> ("String"=w182:string)  [unwired: 9 in]
      n128 = Concatenate Strings(w182, w179) -> (w184:string)
    }
    frame "ALCR" {
      n129 = call "FGV-Funktionstasten.vi"("Aktion"=Funktionstasten-Aktion."Lesen") -> ("Busy"=w255:bool)  [unwired: 7 in, 7 out]
      n130 = case shown="False" w255 {
        tunnel: w252 -> [w265 w306]
        tunnel: [w262 w305] -> w253
        tunnel: w254 -> [w263 _]
        frame False {
          n131 = Index Array(array=w263, index #1=1 ("Index"), index #2=2 ("Index"), index #3=3 ("Index")) -> (element #1=w261:string, element #2=w259:string, element #3=w257:string)
          n132 = case shown="\"KV\"" w261 {
            tunnel: w265 -> [w269 w303]
            tunnel: [w268 w302] -> w262
            tunnel: w259 -> [w267 _]
            tunnel: w257 -> [w266 _]
            frame "KV" {
              n133 = case shown="\"L1\"" w267 {
                tunnel: w269 -> [w271 w297]
                tunnel: [w270 w295] -> w268
                tunnel: w266 -> [_ w296]
                frame "False", Default {
                  n134 = call "Zustandsfehlerinformation.vi"("Aktionen"=Aktionen_Zustandsfehlerinformation."Syntax Error", "String"=w271) -> ("String"=w270:string)  [unwired: 9 in]
                }
                frame "L1" {
                  n135 = call "Protokolldaten_leak check.vi"("Aktion"=Aktion_Protokolldaten_Leak_check."lesen") -> ("Start"=w291:timestamp, "Auswertung"=w289:string[], "Daten"=w275:T38)  [unwired: 23 in, 1 out]
                  n136 = Equal?(x=w296, y="Z") -> (x = y?=w287:bool)
                  n137 = case shown="True" w287 {
                    tunnel: w291 -> [_ w301]
                    tunnel: [_ w299] -> w279
                    tunnel: [_ w298] -> w280
                    frame False {
                    }
                    frame True {
                      n138 = Format Date/Time String(time format string (%c)="%Y%m%d %H%M%S" ("Zeitformatierungs-String (%c)"), seconds (now)=w301) -> (date/time string=w299:string)  [unwired: 1 in]
                      n139 = call <vilib>:"Space Constant.vi"() -> ("String"=w298:string)
                    }
                  }
                  n140 = Unbundle By Name(w275) -> ("Ergebnis mol/s"=w274:sgl, "Leak in %"=w273:sgl)
                  n141 = call "Zustandsfehlerinformation.vi"("Aktionen"=Aktionen_Zustandsfehlerinformation."OK", "String"=w297) -> ("String"=w284:string)  [unwired: 9 in]
                  n142 = Array Size(array=w289) -> (size(s)=w290:i32)
                  n143 = Decrement(x=w290) -> (x-1=w288:i32)
                  n144 = Index Array(array=w289, index=w288) -> (element=w283:string)
                  n145 = Number To Fractional String(number=w274, precision (6)=i16 12 ("Genauigkeit (6)")) -> ()  [unwired: 2 in, 1 out]
                  n146 = Number To Fractional String(number=w273, precision (6)=i16 3 ("Genauigkeit (6)")) -> (F-format string=w277:string)  [unwired: 2 in]
                  n147 = Number To Fractional String(number=0.5 ("Zahl"), precision (6)=i16 3 ("Genauigkeit (6)")) -> (F-format string=w282:string)  [unwired: 2 in]
                  n148 = call <vilib>:"Space Constant.vi"() -> ("String"=w281:string)
                  n149 = Concatenate Strings(w284, w281, w283, w281, w277, w281, w282, w280, w279) -> (w295:string)
                }
              }
            }
            frame "False", Default {
              n150 = call "Zustandsfehlerinformation.vi"("Aktionen"=Aktionen_Zustandsfehlerinformation."Syntax Error", "String"=w303) -> ("String"=w302:string)  [unwired: 9 in]
            }
          }
        }
        frame True {
          n151 = call "Zustandsfehlerinformation.vi"("Aktionen"=Aktionen_Zustandsfehlerinformation."Busy", "String"=w306) -> ("String"=w305:string)  [unwired: 9 in]
        }
      }
    }
    frame "ALEC" {
      n152 = call "Zustandsfehlerinformation.vi"("Aktionen"=Aktionen_Zustandsfehlerinformation."OK", "String"=w321) -> ("String"=w320:string)  [unwired: 9 in]
      n153 = call "Status Dichtheitstest.vi"("Aktionen"=Status_Dichtheitstest_Aktionen."lesen") -> ("Fehler"=w309:bool, "läuft?"=w313:bool, "Anstieg"=w318:sgl)  [unwired: 6 in, 2 out]
      n154 = Or(x=w313, y=w309) -> (x .or. y?=w312:bool)
      n155 = Number To Decimal String(number=w318) -> (decimal integer string=w317:string)  [unwired: 1 in]
      n156 = call <vilib>:"Space Constant.vi"() -> ("String"=w316:string)
      n157 = Concatenate Strings(w320, w316, w317) -> (w315:string)
      n158 = Select(t="error", s=w309, f="busy") -> (s? t:f=w308:string)
      n159 = case shown="True" w312 {
        tunnel: w315 -> [w323 w326]
        tunnel: [w323 w324] -> w314
        tunnel: w308 -> [_ w325]
        frame False {
        }
        frame True {
          n160 = call <vilib>:"Space Constant.vi"() -> ("String"=w327:string)
          n161 = Concatenate Strings(w326, w327, w325) -> (w324:string)
        }
      }
    }
    frame "ALES" {
      n162 = call "FGV Erweiterte Konfig.vi"("Aktion"=FGV_PID_Aktionen."Lesen") -> ("Sonstige"=w334:T39)  [unwired: 5 in, 5 out]
      n163 = call "Zustandsfehlerinformation.vi"("Aktionen"=Aktionen_Zustandsfehlerinformation."OK", "String"=w342) -> ("String"=w339:string)  [unwired: 9 in]
      n164 = Unbundle By Name(w334) -> ("Dichtheitstest Zeit"=w331:sgl, "Dichtheitstest Abfall"=w330:sgl, "Dichtheitstest Umfang"=w329:T42)
      n165 = Number To Fractional String(number=w331, precision (6)=i16 0 ("Genauigkeit (6)")) -> (F-format string=w328:string)  [unwired: 2 in]
      n166 = Number To Fractional String(number=w330, precision (6)=i16 0 ("Genauigkeit (6)")) -> (F-format string=w335:string)  [unwired: 2 in]
      n167 = Number To Fractional String(number=w329, precision (6)=i16 0 ("Genauigkeit (6)")) -> (F-format string=w336:string)  [unwired: 2 in]
      n168 = Build Array(w328, w335, w336) -> (w341:string[])
      n169 = for {
        tunnel: w341 -> [w344] mode=indexing
        shift-right: [w345] -> w340
        shift-left: w339 -> [w347]
        n170 = call <vilib>:"Space Constant.vi"() -> ("String"=w346:string)
        n171 = Concatenate Strings(w347, w346, w344) -> (w345:string)
      }
    }
    frame "ALNB" {
      n172 = call "Zustandsfehlerinformation.vi"("Aktionen"=Aktionen_Zustandsfehlerinformation."OK", "String"=w354) -> ("String"=w353:string)  [unwired: 9 in]
      n173 = call "FGV Erweiterte Konfig.vi"("Aktion"=FGV_PID_Aktionen."Lesen") -> ("Sonstige"=w350:T39)  [unwired: 5 in, 5 out]
      n174 = Unbundle By Name(w350) -> ("Befüllung aktiv"=w348:T41)
      n175 = call <vilib>:"Space Constant.vi"() -> ("String"=w352:string)
      n176 = Number To Decimal String(number=w348) -> (decimal integer string=w351:string)  [unwired: 1 in]
      n177 = Concatenate Strings(w353, w352, w351) -> (w356:string)
    }
    frame "ANOS" {
      n178 = call "Zustandsfehlerinformation.vi"("Aktionen"=Aktionen_Zustandsfehlerinformation."OK", "String"=w362) -> ("String"=w361:string)  [unwired: 9 in]
      n179 = call "FGV FT-IR Parameter.vi"("Aktion"=FGV_FT-IR_Aktionen."lesen") -> ("NoOfScan"=w357:u32)  [unwired: 11 in, 7 out]
      n180 = call <vilib>:"Space Constant.vi"() -> ("String"=w360:string)
      n181 = Number To Decimal String(number=w357) -> (decimal integer string=w359:string)  [unwired: 1 in]
      n182 = Concatenate Strings(w361, w360, w359) -> (w364:string)
    }
    frame "ARCP" {
      n183 = call "Zustandsfehlerinformation.vi"("Aktionen"=Aktionen_Zustandsfehlerinformation."OK", "String"=w369) -> ("String"=w368:string)  [unwired: 9 in]
      n184 = call "FGV FT-IR Parameter.vi"("Aktion"=FGV_FT-IR_Aktionen."lesen") -> ("Current Recipe"=w365:string)  [unwired: 11 in, 7 out]
      n185 = call <vilib>:"Space Constant.vi"() -> ("String"=w367:string)
      n186 = Concatenate Strings(w368, w367, w365) -> (w371:string)
    }
    frame "ARLT" {
      # "#ARLT Rezptliste wie bei MKS"
      n187 = disable-structure shown="Aktiviert" {
        disable-tunnel: w386 -> [w388 w390]
        disable-tunnel: [w387 w390] -> w374
        frame Disabled {
          n188 = call "Zustandsfehlerinformation.vi"("Aktionen"=Aktionen_Zustandsfehlerinformation."OK", "String"=w388) -> ("String"=w387:string)  [unwired: 9 in]
        }
        frame Enabled {
        }
      }
      n189 = call "FGV Rezepte wechseln.vi"("Aktion"=Aktion_FGV_Rezepte_wechseln."lesen") -> ("Rezepte"=w375:string[])  [unwired: 8 in, 6 out]
      n190 = Array To Spreadsheet String(delimiter (Tab)="],[" ("Trennzeichen (Tabulator)"), array=w375, 3:"%s" ("Format-String")) -> (spreadsheet string=w384:string)
      n191 = String Length(string=w384) -> (length=w381:i32)
      n192 = Subtract(x=w381, y=2) -> (x-y=w383:i32)
      n193 = String Subset(string=w384, length (rest)=w383) -> (substring=w379:string)  [unwired: 1 in]
      n194 = call <vilib>:"Space Constant.vi"() -> ("String"=w372:string)
      n195 = Concatenate Strings(w374, w372, "\"[" ("String"), w379, "]\"") -> (w373:string)
    }
    frame "AGSL" {
      # "#AGLB Gasliste wie bei MKS"
      n196 = call "Zustandsfehlerinformation.vi"("Aktionen"=Aktionen_Zustandsfehlerinformation."OK", "String"=w410) -> ("String"=w400:string)  [unwired: 9 in]
      n197 = call "FGV FT-IR Parameter.vi"("Aktion"=FGV_FT-IR_Aktionen."lesen") -> ("NoOfGasses"=w395:u32)  [unwired: 11 in, 7 out]
      n198 = call "FGV Gasliste.vi"("Aktionen"=FGV_FT-IR_Gasliste_Aktionen."lesen") -> ("Aktuelle Gasliste FT-IR"=w393:T36[])  [unwired: 8 in, 2 out]
      n199 = Delete From Array(array=w393, length=w395, index=0 ("Index")) -> (deleted portion=w392:T36[])  [unwired: 1 out]
      n200 = Array To Spreadsheet String(delimiter (Tab)="\" \"" ("Trennzeichen (Tabulator)"), array=w392, 3:"%s" ("Format-String")) -> (spreadsheet string=w409:string)
      n201 = String Length(string=w409) -> (length=w406:i32)
      n202 = Subtract(x=w406, y=2) -> (x-y=w408:i32)
      n203 = String Subset(string=w409, length (rest)=w408) -> (substring=w404:string)  [unwired: 1 in]
      n204 = call <vilib>:"Space Constant.vi"() -> ("String"=w398:string)
      n205 = Concatenate Strings(w400, w398, "\"" ("String"), w404, "\"") -> (w399:string)
    }
    frame "AGSO" {
      w413 = 2 ("y")
      # "AGSO wird an MKS weitergeleitet und die Antwort ausgegeben"
      n206 = call <vilib>:"Space Constant.vi"() -> ("String"=w427:string)
      n207 = Array To Spreadsheet String(delimiter (Tab)=w427, array=w425, 3:"%s" ("Format-String")) -> (spreadsheet string=w411:string)
      n208 = String Length(string=w411) -> (length=w415:i32)
      n209 = Subtract(x=w415, y=w413) -> (x-y=w414:i32)
      n210 = call "Zustandsfehlerinformation.vi"("Aktionen"=Aktionen_Zustandsfehlerinformation."OK", "String"=w420) -> ("String"=w419:string)  [unwired: 9 in]
      n211 = Replace Substring(2:w413, 3:w414, 5:w411) -> (1:w412:string)  [unwired: 1 in, 1 out]
      n212 = call "FGV SGSF und SGSO weiterleiten.vi"("Aktion"=Aktion_FGV_SGSF_und_SGSO_weiterleiten."AGSO löschen") -> ("error out"=w424:errorcluster)  [unwired: 6 in, 8 out]
      n213 = flat-sequence {
        tunnel: w412 -> [w443]
        tunnel: w424 -> [_]
        tunnel: [w441] -> w423
        frame #0 {
          n214 = call "Kommandos verwalten.vi"("Aktionen"=Kommandos_verwalten_Aktionen."setzen Pos1", "neues Kommando"=w443) -> ("NEUE Kommandos"=w441:string[])  [unwired: 7 in, 2 out]
        }
      }
      n215 = Get Date/Time In Seconds() -> (seconds since 1Jan1904=w422:timestamp)
      n216 = while {
        tunnel: w423 -> [_]
        shift-right: [w437] -> _
        shift-left: w422 -> [w437]
        tunnel: [w432] -> w421
        tunnel: [w431] -> w417
        stop <- w434 stop-if-true
        n217 = Get Date/Time In Seconds() -> (seconds since 1Jan1904=w438:timestamp)
        n218 = Wait Until Next ms Multiple(millisecond multiple=u32 10 ("ms")) -> ()  [unwired: 1 out]
        n219 = Subtract(x=w438, y=w437) -> (x-y=w436:dbl)
        n220 = call "FGV SGSF und SGSO weiterleiten.vi"("Aktion"=Aktion_FGV_SGSF_und_SGSO_weiterleiten."lesen") -> ("AGSO"=w431:string, "AGSO aktuell"=w432:bool)  [unwired: 6 in, 7 out]
        n221 = Greater Or Equal?(x=w436, y=3.0) -> (x >= y?=w433:bool)
        n222 = Or(x=w433, y=w432) -> (x .or. y?=w434:bool)
      }
      n223 = case shown="True" w421 {
        frame False {
        }
        frame True {
          n224 = call "FGV SGSF und SGSO weiterleiten.vi"("Aktion"=Aktion_FGV_SGSF_und_SGSO_weiterleiten."AGSO löschen") -> ()  [unwired: 6 in, 9 out]
        }
      }
      n225 = call <vilib>:"Space Constant.vi"() -> ("String"=w418:string)
      n226 = Concatenate Strings(w419, w418, w417) -> (w416:string)
    }
    frame "SGSF" {
      w446 = 2 ("y")
      # "SGSF wird an MKS weitergeleitet und die Antwort ausgegeben"
      n227 = call <vilib>:"Space Constant.vi"() -> ("String"=w460:string)
      n228 = Array To Spreadsheet String(delimiter (Tab)=w460, array=w458, 3:"%s" ("Format-String")) -> (spreadsheet string=w444:string)
      n229 = String Length(string=w444) -> (length=w448:i32)
      n230 = Subtract(x=w448, y=w446) -> (x-y=w447:i32)
      n231 = call "Zustandsfehlerinformation.vi"("Aktionen"=Aktionen_Zustandsfehlerinformation."OK", "String"=w453) -> ("String"=w452:string)  [unwired: 9 in]
      n232 = Replace Substring(2:w446, 3:w447, 5:w444) -> (1:w445:string)  [unwired: 1 in, 1 out]
      n233 = call "FGV SGSF und SGSO weiterleiten.vi"("Aktion"=Aktion_FGV_SGSF_und_SGSO_weiterleiten."SGSF löschen") -> ("error out"=w457:errorcluster)  [unwired: 6 in, 8 out]
      n234 = flat-sequence {
        tunnel: w445 -> [w476]
        tunnel: w457 -> [_]
        tunnel: [w474] -> w456
        frame #0 {
          n235 = call "Kommandos verwalten.vi"("Aktionen"=Kommandos_verwalten_Aktionen."setzen Pos1", "neues Kommando"=w476) -> ("NEUE Kommandos"=w474:string[])  [unwired: 7 in, 2 out]
        }
      }
      n236 = Get Date/Time In Seconds() -> (seconds since 1Jan1904=w455:timestamp)
      n237 = while {
        tunnel: w456 -> [_]
        shift-right: [w470] -> _
        shift-left: w455 -> [w470]
        tunnel: [w464] -> w454
        tunnel: [w465] -> w450
        stop <- w467 stop-if-true
        n238 = Get Date/Time In Seconds() -> (seconds since 1Jan1904=w471:timestamp)
        n239 = Wait Until Next ms Multiple(millisecond multiple=u32 10 ("ms")) -> ()  [unwired: 1 out]
        n240 = Subtract(x=w471, y=w470) -> (x-y=w469:dbl)
        n241 = call "FGV SGSF und SGSO weiterleiten.vi"("Aktion"=Aktion_FGV_SGSF_und_SGSO_weiterleiten."lesen") -> ("SGSF aktuell"=w464:bool, "SGSF"=w465:string)  [unwired: 6 in, 7 out]
        n242 = Greater Or Equal?(x=w469, y=3.0) -> (x >= y?=w466:bool)
        n243 = Or(x=w466, y=w464) -> (x .or. y?=w467:bool)
      }
      n244 = case shown="True" w454 {
        frame False {
        }
        frame True {
          n245 = call "FGV SGSF und SGSO weiterleiten.vi"("Aktion"=Aktion_FGV_SGSF_und_SGSO_weiterleiten."SGSF löschen") -> ()  [unwired: 6 in, 9 out]
        }
      }
      n246 = call <vilib>:"Space Constant.vi"() -> ("String"=w451:string)
      n247 = Concatenate Strings(w452, w451, w450) -> (w449:string)
    }
    frame "SGSO" {
      w479 = 2 ("y")
      # "SGSF wird an MKS weitergeleitet und die Antwort ausgegeben"
      n248 = call <vilib>:"Space Constant.vi"() -> ("String"=w493:string)
      n249 = Array To Spreadsheet String(delimiter (Tab)=w493, array=w491, 3:"%s" ("Format-String")) -> (spreadsheet string=w477:string)
      n250 = String Length(string=w477) -> (length=w481:i32)
      n251 = Subtract(x=w481, y=w479) -> (x-y=w480:i32)
      n252 = call "Zustandsfehlerinformation.vi"("Aktionen"=Aktionen_Zustandsfehlerinformation."OK", "String"=w486) -> ("String"=w485:string)  [unwired: 9 in]
      n253 = Replace Substring(2:w479, 3:w480, 5:w477) -> (1:w478:string)  [unwired: 1 in, 1 out]
      n254 = call "FGV SGSF und SGSO weiterleiten.vi"("Aktion"=Aktion_FGV_SGSF_und_SGSO_weiterleiten."SGSO löschen") -> ("error out"=w490:errorcluster)  [unwired: 6 in, 8 out]
      n255 = flat-sequence {
        tunnel: w478 -> [w509]
        tunnel: w490 -> [_]
        tunnel: [w507] -> w489
        frame #0 {
          n256 = call "Kommandos verwalten.vi"("Aktionen"=Kommandos_verwalten_Aktionen."setzen Pos1", "neues Kommando"=w509) -> ("NEUE Kommandos"=w507:string[])  [unwired: 7 in, 2 out]
        }
      }
      n257 = Get Date/Time In Seconds() -> (seconds since 1Jan1904=w488:timestamp)
      n258 = while {
        tunnel: w489 -> [_]
        shift-right: [w503] -> _
        shift-left: w488 -> [w503]
        tunnel: [w497] -> w487
        tunnel: [w498] -> w483
        stop <- w500 stop-if-true
        n259 = Get Date/Time In Seconds() -> (seconds since 1Jan1904=w504:timestamp)
        n260 = Wait Until Next ms Multiple(millisecond multiple=u32 10 ("ms")) -> ()  [unwired: 1 out]
        n261 = Subtract(x=w504, y=w503) -> (x-y=w502:dbl)
        n262 = call "FGV SGSF und SGSO weiterleiten.vi"("Aktion"=Aktion_FGV_SGSF_und_SGSO_weiterleiten."lesen") -> ("SGSO aktuell"=w497:bool, "SGSO"=w498:string)  [unwired: 6 in, 7 out]
        n263 = Greater Or Equal?(x=w502, y=3.0) -> (x >= y?=w499:bool)
        n264 = Or(x=w499, y=w497) -> (x .or. y?=w500:bool)
      }
      n265 = case shown="True" w487 {
        frame False {
        }
        frame True {
          n266 = call "FGV SGSF und SGSO weiterleiten.vi"("Aktion"=Aktion_FGV_SGSF_und_SGSO_weiterleiten."SGSO löschen") -> ()  [unwired: 6 in, 9 out]
        }
      }
      n267 = call <vilib>:"Space Constant.vi"() -> ("String"=w484:string)
      n268 = Concatenate Strings(w485, w484, w483) -> (w482:string)
    }
    frame "AGSF" {
      w512 = 2 ("y")
      # "AGSF wird an MKS weitergeleitet und die Antwort ausgegeben"
      n269 = call <vilib>:"Space Constant.vi"() -> ("String"=w526:string)
      n270 = Array To Spreadsheet String(delimiter (Tab)=w526, array=w524, 3:"%s" ("Format-String")) -> (spreadsheet string=w511:string)
      n271 = String Length(string=w511) -> (length=w514:i32)
      n272 = Subtract(x=w514, y=w512) -> (x-y=w513:i32)
      n273 = call "Zustandsfehlerinformation.vi"("Aktionen"=Aktionen_Zustandsfehlerinformation."OK", "String"=w519) -> ("String"=w518:string)  [unwired: 9 in]
      n274 = Replace Substring(2:w512, 3:w513, 5:w511) -> (1:w510:string)  [unwired: 1 in, 1 out]
      n275 = call "FGV SGSF und SGSO weiterleiten.vi"("Aktion"=Aktion_FGV_SGSF_und_SGSO_weiterleiten."AGSF löschen") -> ("error out"=w523:errorcluster)  [unwired: 6 in, 8 out]
      n276 = flat-sequence {
        tunnel: w523 -> [_]
        tunnel: [w541] -> w522
        tunnel: w510 -> [w540]
        frame #0 {
          n277 = call "Kommandos verwalten.vi"("Aktionen"=Kommandos_verwalten_Aktionen."setzen Pos1", "neues Kommando"=w540) -> ("NEUE Kommandos"=w541:string[])  [unwired: 7 in, 2 out]
        }
      }
      n278 = Get Date/Time In Seconds() -> (seconds since 1Jan1904=w521:timestamp)
      n279 = while {
        tunnel: w522 -> [_]
        shift-right: [w536] -> _
        shift-left: w521 -> [w536]
        tunnel: [w530] -> w520
        tunnel: [w531] -> w516
        stop <- w533 stop-if-true
        n280 = Get Date/Time In Seconds() -> (seconds since 1Jan1904=w537:timestamp)
        n281 = Wait Until Next ms Multiple(millisecond multiple=u32 10 ("ms")) -> ()  [unwired: 1 out]
        n282 = Subtract(x=w537, y=w536) -> (x-y=w535:dbl)
        n283 = call "FGV SGSF und SGSO weiterleiten.vi"("Aktion"=Aktion_FGV_SGSF_und_SGSO_weiterleiten."lesen") -> ("AGSF"=w531:string, "AGSF aktuell"=w530:bool)  [unwired: 6 in, 7 out]
        n284 = Greater Or Equal?(x=w535, y=3.0) -> (x >= y?=w532:bool)
        n285 = Or(x=w532, y=w530) -> (x .or. y?=w533:bool)
      }
      n286 = case shown="True" w520 {
        frame False {
        }
        frame True {
          n287 = call "FGV SGSF und SGSO weiterleiten.vi"("Aktion"=Aktion_FGV_SGSF_und_SGSO_weiterleiten."AGSF löschen") -> ()  [unwired: 6 in, 9 out]
        }
      }
      n288 = call <vilib>:"Space Constant.vi"() -> ("String"=w517:string)
      n289 = Concatenate Strings(w518, w517, w516) -> (w515:string)
    }
    frame "ASBE" {
      n290 = call "Zustandsfehlerinformation.vi"("Aktionen"=Aktionen_Zustandsfehlerinformation."OK", "String"=w548) -> ("String"=w547:string)  [unwired: 9 in]
      n291 = call "FGV FT-IR Parameter.vi"("Aktion"=FGV_FT-IR_Aktionen."lesen") -> ("Ausgangs-Cluster"=w544:T43)  [unwired: 11 in, 7 out]
      n292 = Unbundle By Name(w544) -> ("(82) labBaseName"=w543:string)
      n293 = call <vilib>:"Space Constant.vi"() -> ("String"=w546:string)
      n294 = Concatenate Strings(w547, w546, w543) -> (w550:string)
    }
    frame "ASLO" {
      n295 = call "FGV FT-IR Parameter.vi"("Aktion"=FGV_FT-IR_Aktionen."lesen") -> ("Ausgangs-Cluster"=w553:T43)  [unwired: 11 in, 7 out]
      n296 = call "Zustandsfehlerinformation.vi"("Aktionen"=Aktionen_Zustandsfehlerinformation."OK", "String"=w558) -> ("String"=w557:string)  [unwired: 9 in]
      n297 = Unbundle By Name(w553) -> ("Spektrum loggen aktiv?"=w552:bool)
      n298 = Boolean To (0,1)(Boolean=w552) -> (0, 1=w551:i16)
      n299 = call <vilib>:"Space Constant.vi"() -> ("String"=w555:string)
      n300 = Number To Decimal String(number=w551) -> (decimal integer string=w556:string)  [unwired: 1 in]
      n301 = Concatenate Strings(w557, w555, w556) -> (w560:string)
    }
    frame "ASNR" {
      n302 = call "FGV FT-IR Parameter.vi"("Aktion"=FGV_FT-IR_Aktionen."lesen") -> ("Ausgangs-Cluster"=w562:T43)  [unwired: 11 in, 7 out]
      n303 = call "Zustandsfehlerinformation.vi"("Aktionen"=Aktionen_Zustandsfehlerinformation."OK", "String"=w566) -> ("String"=w565:string)  [unwired: 9 in]
      n304 = Unbundle By Name(w562) -> ("(83) labIndex"=w561:string)
      n305 = call <vilib>:"Space Constant.vi"() -> ("String"=w564:string)
      n306 = Concatenate Strings(w565, w564, w561) -> (w568:string)
    }
    frame "ASTF" {
      n307 = call "Zustandsfehlerinformation.vi"("Aktionen"=Aktionen_Zustandsfehlerinformation."OK", "String"=w573) -> ("String"=w572:string)  [unwired: 9 in]
      n308 = call "Fehler Zaehler.vi"("Aktionen"=Aktionen_Stoernummern_pruefen."lesen") -> ("Fehler Nummern"=w570:string)  [unwired: 7 in, 3 out]
      n309 = call <vilib>:"Space Constant.vi"() -> ("String"=w569:string)
      n310 = Concatenate Strings(w572, w569, w570) -> (w575:string)
    }
    frame "ASTZ" {
      n311 = call "Zustandsfehlerinformation.vi"("Aktionen"=Aktionen_Zustandsfehlerinformation."OK", "String"=w585) -> ("String"=w584:string)  [unwired: 9 in]
      n312 = call "FGV Schedule Status.vi"("Aktion"=Aktion_FGV_Scheduler_Status."lesen") -> ("Scheduler Status"=w578:bool)  [unwired: 13 in, 1 out]
      n313 = call "FGV-Funktionstasten.vi"("Aktion"=Funktionstasten-Aktion."Lesen") -> ("ausgewählte Funktion"=w577:T12, "Betriebsart"=w582:T22)  [unwired: 7 in, 6 out]
      n314 = case shown="True" w578 {
        tunnel: w577 -> [w589 _]
        tunnel: [w588 "SATK" ("String")] -> w576
        frame False {
          n315 = case shown="\"Init 4\"" w589 {
            tunnel: ["STBY" ("String") "SPAU" ("String") "SECO" ("String") "SMGA" ("String") "SATK" ("String") "SEKA" ("String") "SRUC" ("String") "SSPL" ("String") "SNGA" ("String") "SCZP" ("String") _ _ _ _ _ _ _ _] -> w588
            frame "Standby", Default {
            }
            frame "Pause" {
            }
            frame "Eco" {
            }
            frame "Messen" {
            }
            frame "Kalibrieren" {
            }
            frame "Cal-Gas" {
              # "#KaliAutoMessenBug"
            }
            frame "Spülen Filter" {
            }
            frame "Spülen Leitung" {
            }
            frame "0-Gas" {
            }
            frame "CG zu PNS" {
              # "#KaliAutoMessenBug"
            }
            frame "Init 1" {
            }
            frame "Init 2" {
            }
            frame "-------------" {
            }
            frame "Init 3" {
            }
            frame "Init 4" {
            }
            frame "Messen vorbereiten" {
            }
            frame "Messen durchführen" {
            }
            frame "Exit" {
            }
          }
        }
        frame True {
        }
      }
      n316 = case shown="\"Bitparallel\"" w582 {
        tunnel: ["SMAN" ("String") "SREM" ("String") "SBIT" ("String")] -> w581
        frame "Manuell", Default {
        }
        frame "Remote" {
        }
        frame "Bitparallel" {
        }
      }
      n317 = call <vilib>:"Space Constant.vi"() -> ("String"=w580:string)
      n318 = Concatenate Strings(w584, w580, w581, w580, w576) -> (w587:string)
    }
    frame "ATEM" {
      n319 = call "Zustandsfehlerinformation.vi"("Aktionen"=Aktionen_Zustandsfehlerinformation."OK", "String"=w627) -> ("String"=w619:string)  [unwired: 9 in]
      n320 = call "FGV cRIO-Daten.vi"("Aktion"=enum16{"lesen", "schreiben"}."lesen") -> ("TC Eingänge"=w604:T44)  [unwired: 9 in, 9 out]
      n321 = call "FGV PNS Istwerte.vi"("Aktionen"=Aktionen_FGV_Istwerte."lesen") -> ("Regler"=w611:T45)  [unwired: 11 in, 3 out]
      n322 = Unbundle By Name(w604) -> ("TC0: Reserve"=w624:sgl, "TC1: HL zu FT-IR"=w623:sgl, "TC2: HL Extern SP1"=w622:sgl, "TC3: HL Extern SP2"=w618:sgl, "TC4: Reserve"=w617:sgl, "TC5: Reserve"=w616:sgl, "TC6: Reserve"=w615:sgl, "TC7: Reserve"=w614:sgl, "TC8: FT-IR"=w613:sgl)
      n323 = Index Array(array=w611) -> (element #1=w610:T46, element #2=w608:T46, element #3=w607:T46)  [unwired: 3 in]
      n324 = call "FGV FT-IR Diagnosewerte.vi"("Aktionen"=FGV_FT-IR_Diagnose_Aktionen."Lesen") -> ()  [unwired: 5 in, 6 out]
      n325 = Unbundle By Name(w610) -> ("Istwert"=w609:i16)
      n326 = Unbundle By Name(w608) -> ("Istwert"=w606:i16)
      n327 = Unbundle By Name(w607) -> ("Istwert"=w605:i16)
      n328 = Build Array(w624, w623, w622, w618, w617, w616, w615, w614, w613, w609, w606, w605) -> (w621:sgl[])
      n329 = for {
        tunnel: w621 -> [w635] mode=indexing
        shift-right: [w630] -> w620
        shift-left: w619 -> [w633]
        n330 = Number To Fractional String(use system decimal point (T)=FALSE ("Systemdezimalzeichen verwenden (T)"), number=w635, precision (6)=i16 1 ("Genauigkeit (6)")) -> (F-format string=w631:string)  [unwired: 1 in]
        n331 = call <vilib>:"Space Constant.vi"() -> ("String"=w632:string)
        n332 = Concatenate Strings(w633, w632, w631) -> (w630:string)
      }
    }
    frame "AVER" {
      n333 = call "Zustandsfehlerinformation.vi"("Aktionen"=Aktionen_Zustandsfehlerinformation."OK", "String"=w642) -> ("String"=w639:string)  [unwired: 9 in]
      n334 = call "FGV System Konstanten.vi"("Aktionen"=Aktioen_FGV_System_Konstanten."lesen") -> ("Cluster out"=w637:T35)  [unwired: 6 in, 4 out]
      n335 = Unbundle By Name(w637) -> ("Software Version"=w636:string)
      n336 = call <vilib>:"Space Constant.vi"() -> ("String"=w641:string)
      n337 = Concatenate Strings(w639, w641, w636) -> (w638:string)
    }
    frame "EKFG" {
      n338 = Index Array(array=w651, index=1 ("Index")) -> (element=w647:string)
      n339 = Equal?(x=w647, y="K0") -> (x = y?=w645:bool)
      n340 = case shown="True" w645 {
        tunnel: w651 -> [_ w656]
        tunnel: [Aktionen_Zustandsfehlerinformation."Syntax Error" ("Aktionen") w653] -> w644
        frame False {
          # "Befehlskomando NICHT KORREKT!"
        }
        frame True {
          n341 = Delete From Array(array=w656, length=2 ("Länge"), index=0 ("Index")) -> (array with subset deleted=w655:string[])  [unwired: 1 out]
          n342 = Empty Array?(array=w655) -> (empty?=w654:bool)
          n343 = case shown="False" w654 {
            tunnel: w655 -> [w664 _]
            tunnel: [Aktionen_Zustandsfehlerinformation."OK" ("Aktionen") Aktionen_Zustandsfehlerinformation."Datenfehler" ("Aktionen")] -> w653
            frame False {
              n344 = call "AK Namen.vi"("Aktionen"=AK_Namen_Aktionen."EKFG schreiben", "EKFG Liste"=w664) -> ("AK Namen"=w661:string[])  [unwired: 6 in, 3 out]
              n345 = call "AK Namen.vi"("Aktionen"=AK_Namen_Aktionen."EKFG erstellen", "AK Namen"=w661) -> ("AK Namen"=w659:string[])  [unwired: 6 in, 3 out]
              n346 = call "AK Namen.vi"("Aktionen"=AK_Namen_Aktionen."speichern EKFG", "AK Namen"=w659) -> ()  [unwired: 6 in, 4 out]
            }
            frame True {
              # "Fehler mit den Einstell Kommandos"
            }
          }
        }
      }
      n347 = call "Zustandsfehlerinformation.vi"("Aktionen"=w644, "String"=w650) -> ("String"=w649:string)  [unwired: 9 in]
    }
    frame "SATK" {
      n348 = call "Setze Zustand.vi"("AK Befehl"=w668, "Zustand"=Zustaende."Kalibrieren") -> ("Antwort String"=w667:string)  [unwired: 8 in, 1 out]
    }
    frame "SDFT" {
      n349 = call "FGV-Funktionstasten.vi"("Aktion"=Funktionstasten-Aktion."Lesen") -> ("Betriebsart"=w676:T22)  [unwired: 7 in, 7 out]
      n350 = Equal?(x=w676, y=Betriebsart."Remote" ("Betriebsart")) -> (x = y?=w670:bool)
      n351 = case shown="True" w670 {
        tunnel: w673 -> [w678 w691]
        tunnel: [w677 w690] -> w672
        tunnel: w671 -> [_ w689]
        frame False {
          n352 = call "Zustandsfehlerinformation.vi"("Aktionen"=Aktionen_Zustandsfehlerinformation."Offline", "String"=w678) -> ("String"=w677:string)  [unwired: 9 in]
        }
        frame True {
          n353 = Index Array(array=w689, index=2 ("Index")) -> (element=w680:string)
          n354 = Decimal String To Number(string=w680, default (0L)=sgl 0.0 ("Standard (0 I32)")) -> (number=w685:sgl)  [unwired: 1 in, 1 out]
          n355 = call "FGV Anlagengrenzwerte.vi"("Aktion"=FGV_Anlagengrenzwerte_Aktionen."Lesen") -> ("Anlagen-Grenzwerte Anzeige"=w683:T31)  [unwired: 1 in, 9 out]
          n356 = Bundle By Name(cluster=w683, "Durchfluss FT-IR:.Sollwert"=w685) -> (w684:T31)
          n357 = call "Zustandsfehlerinformation.vi"("Aktionen"=Aktionen_Zustandsfehlerinformation."OK", "String"=w691) -> ("String"=w690:string)  [unwired: 9 in]
          n358 = call "FGV Anlagengrenzwerte.vi"("Aktion"=FGV_Anlagengrenzwerte_Aktionen."Grenzwerte schreiben", "Anlagen-Grenzwerte Anzeige"=w684) -> ()  [unwired: 10 out]
        }
      }
    }
    frame "SGSC" {
      # "1...Gasindex\n2...Sollkonz.\n3....Mittelung in sec"
      # "#SGSC Setze Gas Span über Concentration"
      n359 = Index Array(array=w705, index #1=1 ("Index"), index #2=2 ("Index"), index #3=3 ("Index")) -> (element #1=w699:string, element #2=w696:string, element #3=w694:string)
      n360 = Empty String/Path?(string/path=w694) -> (empty?=w692:bool)
      n361 = Decimal Digit?(1:w694) -> (0:w695:bool)
      n362 = Decimal Digit?(1:w696) -> (0:w697:bool)
      n363 = Decimal Digit?(1:w699) -> (0:w698:bool)
      n364 = Or(x=w695, y=w692) -> (x .or. y?=w693:bool)
      n365 = case shown="True" w698 {
        tunnel: w699 -> [_ w713]
        tunnel: w701 -> [w710 w718]
        tunnel: [w708 w717] -> w700
        tunnel: w697 -> [_ w719]
        tunnel: w696 -> [_ w715]
        tunnel: w693 -> [_ w716]
        tunnel: w694 -> [_ w714]
        tunnel: w692 -> [_ w712]
        frame False {
          # "Gasindex not numerical value"
          n366 = call "Zustandsfehlerinformation.vi"("Aktionen"=Aktionen_Zustandsfehlerinformation."Datenfehler", "String"=w710) -> ("String"=w709:string)  [unwired: 9 in]
          n367 = call <vilib>:"Space Constant.vi"() -> ("String"=w706:string)
          n368 = Concatenate Strings(w709, w706, "1" ("String")) -> (w708:string)
        }
        frame True {
          n369 = case shown="True" w719 {
            tunnel: w718 -> [w721 w732]
            tunnel: [w720 w731] -> w717
            tunnel: w716 -> [_ w730]
            tunnel: w715 -> [_ w729]
            tunnel: w714 -> [_ w728]
            tunnel: w713 -> [_ w727]
            tunnel: w712 -> [_ w726]
            frame False {
              # "Sollwertkonzentration not numerical value"
              n370 = call "Zustandsfehlerinformation.vi"("Aktionen"=Aktionen_Zustandsfehlerinformation."Datenfehler", "String"=w721) -> ("String"=w724:string)  [unwired: 9 in]
              n371 = call <vilib>:"Space Constant.vi"() -> ("String"=w722:string)
              n372 = Concatenate Strings(w724, w722, "3" ("String")) -> (w720:string)
            }
            frame True {
              n373 = case shown="True" w730 {
                tunnel: w732 -> [w734 w742]
                tunnel: [w733 w741] -> w731
                tunnel: w729 -> [_ w749]
                tunnel: w728 -> [_ w752]
                tunnel: w727 -> [_ w751]
                tunnel: w726 -> [_ w739]
                frame False {
                  # "Mittelung keine Zahl"
                  n374 = call "Zustandsfehlerinformation.vi"("Aktionen"=Aktionen_Zustandsfehlerinformation."Datenfehler", "String"=w734) -> ("String"=w737:string)  [unwired: 9 in]
                  n375 = call <vilib>:"Space Constant.vi"() -> ("String"=w735:string)
                  n376 = Concatenate Strings(w737, w735, "5" ("String")) -> (w733:string)
                }
                frame True {
                  n377 = case shown="False" w739 {
                    tunnel: w752 -> [w757 _]
                    tunnel: [w753 u32 1 ("Obergrenze")] -> w740
                    frame False {
                      n378 = Decimal String To Number(string=w757) -> (number=w755:i32)  [unwired: 2 in, 1 out]
                      n379 = In Range and Coerce(upper limit=u32 60 ("Obergrenze"), x=w755, lower limit=u32 1 ("Untergrenze")) -> (coerced(x)=w753:u32)  [unwired: 1 out]
                    }
                    frame True {
                      # "Standardwert 1 sec"
                    }
                  }
                  n380 = Decimal String To Number(string=w751) -> (number=w744:i32)  [unwired: 2 in, 1 out]
                  n381 = Fract/Exp String To Number(use system decimal point (T)=FALSE ("Systemdezimalzeichen verwenden (T)"), string=w749) -> (number=w748:dbl)  [unwired: 2 in, 1 out]
                  n382 = call "FGV FT-IR Parameter.vi"("Aktion"=FGV_FT-IR_Aktionen."lesen") -> ("NoOfGasses"=w746:u32)  [unwired: 11 in, 7 out]
                  n383 = In Range and Coerce(upper limit=w746, x=w744, lower limit=u32 1 ("Untergrenze")) -> (In Range?=w743:bool)  [unwired: 1 out]
                  n384 = case shown="True" w743 {
                    tunnel: w740 -> [_ w769]
                    tunnel: w748 -> [_ w768]
                    tunnel: w744 -> [_ w767]
                    tunnel: w742 -> [w760 w766]
                    tunnel: [w759 w765] -> w741
                    frame False {
                      # "Index out of Range Gasnumber"
                      n385 = call "Zustandsfehlerinformation.vi"("Aktionen"=Aktionen_Zustandsfehlerinformation."Datenfehler", "String"=w760) -> ("String"=w763:string)  [unwired: 9 in]
                      n386 = call <vilib>:"Space Constant.vi"() -> ("String"=w761:string)
                      n387 = Concatenate Strings(w763, w761, "2" ("String")) -> (w759:string)
                    }
                    frame True {
                      n388 = stacked-sequence {
                        seq-local: [w770 _ _ _] -> [_ _ w802 _]
                        seq-local: [_ w785 _ _] -> [_ _ w803 _]
                        seq-local: [_ _ w801 _] -> [_ _ _ w832]
                        seq-local: [_ _ w800 _] -> [_ _ _ w831]
                        tunnel: w769 -> [_ _ w807 _]
                        tunnel: w767 -> [_ _ w806 _]
                        tunnel: w768 -> [_ _ w805 _]
                        tunnel: w766 -> [_ _ _ w834]
                        tunnel: [_ _ _ w833] -> w765
                        frame #0 {
                          n389 = call "Kommandos verwalten.vi"("Aktionen"=Kommandos_verwalten_Aktionen."setzen Pos1", "neues Kommando"="AGSF") -> ("Zeitstempeln"=w772:timestamp[])  [unwired: 7 in, 2 out]
                          n390 = Get Date/Time In Seconds() -> (seconds since 1Jan1904=w771:timestamp)
                          n391 = while {
                            tunnel: w772 -> [_]
                            shift-right: [w777] -> _
                            shift-left: w771 -> [w777]
                            tunnel: [w775] -> w770
                            stop <- w776 stop-if-true
                            n392 = call "FGV Span.vi"("Aktion"=Aktion_FGV_Span."lesen") -> ("Aktualisiert"=w782:bool)  [unwired: 7 in, 3 out]
                            n393 = Get Date/Time In Seconds() -> (seconds since 1Jan1904=w780:timestamp)
                            n394 = Subtract(x=w780, y=w777) -> (x-y=w779:dbl)
                            n395 = Greater Or Equal?(x=w779, y=3.0) -> (x >= y?=w775:bool)
                            n396 = Or(x=w775, y=w782) -> (x .or. y?=w776:bool)
                            n397 = case shown="True" w776 {
                              frame False {
                              }
                              frame True {
                                n398 = call "FGV Span.vi"("Aktion"=Aktion_FGV_Span."Aktualisierung aufheben") -> ()  [unwired: 7 in, 4 out]
                              }
                            }
                            n399 = Wait Until Next ms Multiple(millisecond multiple=u32 10 ("ms")) -> ()  [unwired: 1 out]
                          }
                        }
                        frame #1 {
                          n400 = call "Kommandos verwalten.vi"("Aktionen"=Kommandos_verwalten_Aktionen."setzen Pos1", "neues Kommando"="AGSO") -> ("Zeitstempeln"=w787:timestamp[])  [unwired: 7 in, 2 out]
                          n401 = Get Date/Time In Seconds() -> (seconds since 1Jan1904=w786:timestamp)
                          n402 = while {
                            tunnel: w787 -> [_]
                            shift-right: [w795] -> _
                            shift-left: w786 -> [w795]
                            tunnel: [w790] -> w785
                            stop <- w791 stop-if-true
                            n403 = call "FGV Span.vi"("Aktion"=Aktion_FGV_Span."lesen") -> ("Aktualisiert"=w797:bool)  [unwired: 7 in, 3 out]
                            n404 = Get Date/Time In Seconds() -> (seconds since 1Jan1904=w794:timestamp)
                            n405 = Subtract(x=w794, y=w795) -> (x-y=w793:dbl)
                            n406 = Greater Or Equal?(x=w793, y=3.0) -> (x >= y?=w790:bool)
                            n407 = Or(x=w790, y=w797) -> (x .or. y?=w791:bool)
                            n408 = case shown="True" w791 {
                              frame False {
                              }
                              frame True {
                                n409 = call "FGV Span.vi"("Aktion"=Aktion_FGV_Span."Aktualisierung aufheben") -> ()  [unwired: 7 in, 4 out]
                              }
                            }
                            n410 = Wait Until Next ms Multiple(millisecond multiple=u32 10 ("ms")) -> ()  [unwired: 1 out]
                          }
                        }
                        frame #2 {
                          n411 = Or(x=w802, y=w803) -> (x .or. y?=w804:bool)
                          n412 = case shown="True" w804 {
                            tunnel: w807 -> [w817 _]
                            tunnel: w806 -> [w816 _]
                            tunnel: w805 -> [w815 _]
                            tunnel: [_ TRUE] -> w801
                            tunnel: [w808 _] -> w800
                            frame False {
                              n413 = Decrement(x=w816) -> (x-1=w814:i32)
                              n414 = call "FGV Span.vi"("Aktion"=Aktion_FGV_Span."lesen") -> ("Offset"=w820:sgl[], "Span"=w821:sgl[])  [unwired: 7 in, 2 out]
                              n415 = Index Array(array=w821, index=w814) -> (element=w818:sgl)
                              n416 = Index Array(array=w820, index=w814) -> (element=w819:sgl)
                              n417 = call "Spanwerte aufzeichnen.vi"("Sollwerte"=w815, "Komponente"=w814, "Offset"=w819, "Aktueller Spanfactor"=w818, "Mittelung in sec"=w817) -> ("Spanfaktor"=w813:sgl)  [unwired: 4 in, 6 out]
                              n418 = In Range and Coerce(upper limit=sgl 1.15 ("Obergrenze"), x=w813, lower limit=sgl 0.85 ("Untergrenze")) -> (coerced(x)=w809:sgl, In Range?=w810:bool)
                              n419 = case shown="True" w810 {
                                tunnel: w814 -> [_ w826]
                                tunnel: w809 -> [_ w824]
                                tunnel: [TRUE _] -> w808
                                frame False {
                                }
                                frame True {
                                n420 = Number To Fractional String(use system decimal point (T)=FALSE ("Systemdezimalzeichen verwenden (T)"), number=w824) -> (F-format string=w827:string)  [unwired: 2 in]
                                n421 = Add(x=9000 ("Feedback"), y=w826) -> (x+y=w829:i32)
                                n422 = call "TOOLweb SET.vi"("Wert-String"=w827, "EVID-Nummer"=w829) -> ()  [unwired: 3 in, 3 out]
                                }
                              }
                            }
                            frame True {
                            }
                          }
                        }
                        frame #3 {
                          n423 = case shown="False" w832 {
                            tunnel: w834 -> [w839 w843]
                            tunnel: [w835 w842] -> w833
                            tunnel: w831 -> [_ w841]
                            frame True {
                              # "Operation wurde nicht ausgeführt\nkeine aktuelle Spanfaktoren vorhanden"
                              n424 = call "Zustandsfehlerinformation.vi"("Aktionen"=Aktionen_Zustandsfehlerinformation."Datenfehler", "String"=w839) -> ("String"=w838:string)  [unwired: 9 in]
                              n425 = call <vilib>:"Space Constant.vi"() -> ("String"=w837:string)
                              n426 = Concatenate Strings(w838, w837, "4" ("String")) -> (w835:string)
                            }
                            frame False {
                              n427 = case shown="True" w841 {
                                tunnel: w843 -> [w848 w854]
                                tunnel: [w844 w850] -> w842
                                frame True {
                                n428 = call "Zustandsfehlerinformation.vi"("Aktionen"=Aktionen_Zustandsfehlerinformation."Datenfehler", "String"=w848) -> ("String"=w847:string)  [unwired: 9 in]
                                n429 = call <vilib>:"Space Constant.vi"() -> ("String"=w846:string)
                                n430 = Concatenate Strings(w847, w846, "5" ("String")) -> (w844:string)
                                }
                                frame False {
                                # "Success"
                                n431 = call "Zustandsfehlerinformation.vi"("Aktionen"=Aktionen_Zustandsfehlerinformation."OK", "String"=w854) -> ("String"=w853:string)  [unwired: 9 in]
                                n432 = call <vilib>:"Space Constant.vi"() -> ("String"=w852:string)
                                n433 = Concatenate Strings(w853, w852, "0" ("String")) -> (w850:string)
                                }
                              }
                            }
                          }
                        }
                      }
                    }
                  }
                }
              }
            }
          }
        }
      }
    }
    frame "SECO" {
      n434 = call "Setze Zustand.vi"("AK Befehl"=w858, "Zustand"=Zustaende."Eco") -> ("Antwort String"=w857:string)  [unwired: 8 in, 1 out]
    }
    frame "SEKA" {
      n435 = call "FGV-Funktionstasten.vi"("Aktion"=Funktionstasten-Aktion."Lesen") -> ("Betriebsart"=w863:T22)  [unwired: 7 in, 7 out]
      n436 = Equal?(x=w863, y=Betriebsart."Remote" ("Betriebsart")) -> (x = y?=w864:bool)
      n437 = case shown="True" w864 {
        tunnel: w860 -> [w866 w872]
        tunnel: [w865 w871] -> w859
        frame False {
          n438 = call "Zustandsfehlerinformation.vi"("Aktionen"=Aktionen_Zustandsfehlerinformation."Offline", "String"=w866) -> ("String"=w865:string)  [unwired: 9 in]
        }
        frame True {
          n439 = call "Gespeicherte Werte.vi"("Aktionen"=Aktionen_Gespeicherte_Werte."lesen") -> ("Diverse Werte"=w873:T29)  [unwired: 6 in, 4 out]
          n440 = Unbundle By Name(w873) -> ("Kalibriergaseingang"=w869:i16)
          n441 = disable-structure shown="Aktiviert" {
            disable-tunnel: [w875 _] -> w868
            frame Disabled {
              n442 = call "FGV System.vi"("Aktionen"=Aktioen_FGV_System."lesen") -> ("Optionen"=w875:T37)  [unwired: 12 in, 6 out]
            }
            frame Enabled {
            }
          }
          n443 = case shown="1" w869 {
            selector: w869 -> [_ w878 _ _]
            tunnel: [Zustaende."Standby" ("Zustand") Zustaende."Cal-Gas" ("Zustand") Zustaende."CG zu PNS" ("Zustand") Zustaende."-------------" ("Zustand")] -> w870
            tunnel: w868 -> [_ w879 _ _]
            frame 0, Default {
            }
            frame 1 {
              n444 = disable-structure shown="Deaktiviert" {
                disable-tunnel: w879 -> [w884 _]
                disable-tunnel: w878 -> [w883 _]
                frame Disabled {
                  n445 = Bundle By Name(cluster=w884, "Span Gas Auswahl"=w883) -> (w882:T37)
                  n446 = call "FGV System.vi"("Optionen"=w882, "Aktionen"=Aktioen_FGV_System."Optionen schreiben") -> ("error out"=w881:errorcluster)  [unwired: 11 in, 6 out]
                  n447 = call "FGV System.vi"("error in (no error)"=w881, "Aktionen"=Aktioen_FGV_System."speichern") -> ()  [unwired: 11 in, 7 out]
                }
                frame Enabled {
                }
              }
            }
            frame 2 {
            }
            frame 3 {
            }
          }
          n448 = call "Setze Zustand.vi"("AK Befehl"=w872, "Zustand"=w870) -> ("Antwort String"=w871:string)  [unwired: 8 in, 1 out]
        }
      }
    }
    frame "SEMB" {
      n449 = call "FGV-Funktionstasten.vi"("Aktion"=Funktionstasten-Aktion."Lesen") -> ("Betriebsart"=w894:T22)  [unwired: 7 in, 7 out]
      n450 = Equal?(x=w894, y=Betriebsart."Remote" ("Betriebsart")) -> (x = y?=w895:bool)
      n451 = case shown="True" w895 {
        tunnel: w891 -> [w897 w909]
        tunnel: [w896 w908] -> w890
        tunnel: w889 -> [_ w907]
        frame False {
          n452 = call "Zustandsfehlerinformation.vi"("Aktionen"=Aktionen_Zustandsfehlerinformation."Offline", "String"=w897) -> ("String"=w896:string)  [unwired: 9 in]
        }
        frame True {
          n453 = Index Array(array=w907, index=2 ("Index")) -> (element=w905:string)
          n454 = call "Zustandsfehlerinformation.vi"("Aktionen"=Aktionen_Zustandsfehlerinformation."OK", "String"=w909) -> ("String"=w908:string)  [unwired: 9 in]
          n455 = Decimal String To Number(string=w905, offset=1 ("Offset (0)")) -> (number=w901:i32)  [unwired: 1 in, 1 out]
          n456 = call "Gespeicherte Werte.vi"("Aktionen"=Aktionen_Gespeicherte_Werte."lesen") -> ("Diverse Werte"=w900:T29)  [unwired: 6 in, 4 out]
          n457 = Bundle By Name(cluster=w900, "Kalibriergaseingang"=w901) -> (w899:T29)
          n458 = call "Gespeicherte Werte.vi"("Aktionen"=Aktionen_Gespeicherte_Werte."Diverse", "Diverse Werte"=w899) -> ()  [unwired: 5 in, 5 out]
        }
      }
    }
    frame "SENT" {
      n459 = call "FGV-Funktionstasten.vi"("Aktion"=Funktionstasten-Aktion."Lesen") -> ("Betriebsart"=w916:T22)  [unwired: 7 in, 7 out]
      n460 = Equal?(x=w916, y=Betriebsart."Remote" ("Betriebsart")) -> (x = y?=w917:bool)
      n461 = case shown="True" w917 {
        tunnel: w913 -> [w919 w931]
        tunnel: [w918 w930] -> w912
        tunnel: w911 -> [_ w929]
        frame False {
          n462 = call "Zustandsfehlerinformation.vi"("Aktionen"=Aktionen_Zustandsfehlerinformation."Offline", "String"=w919) -> ("String"=w918:string)  [unwired: 9 in]
        }
        frame True {
          n463 = Index Array(array=w929, index=2 ("Index")) -> (element=w927:string)
          n464 = call "Zustandsfehlerinformation.vi"("Aktionen"=Aktionen_Zustandsfehlerinformation."OK", "String"=w931) -> ("String"=w930:string)  [unwired: 9 in]
          n465 = Decimal String To Number(string=w927) -> (number=w921:i32)  [unwired: 2 in, 1 out]
          n466 = call "FGV-Funktionstasten.vi"("Samplepoint"=w921, "Aktion"=Funktionstasten-Aktion."Samplepoint") -> ()  [unwired: 6 in, 8 out]
          n467 = call "Gespeicherte Werte.vi"("Aktionen"=Aktionen_Gespeicherte_Werte."lesen") -> ("Diverse Werte"=w924:T29)  [unwired: 6 in, 4 out]
          n468 = Bundle By Name(cluster=w924, "SamplePoint"=w921) -> (w923:T29)
          n469 = call "Gespeicherte Werte.vi"("Aktionen"=Aktionen_Gespeicherte_Werte."Diverse", "Diverse Werte"=w923) -> ()  [unwired: 5 in, 5 out]
        }
      }
    }
    frame "SLCR" {
      n470 = Index Array(array=w935, index=1 ("Index")) -> (element=w941:string)
      n471 = call "FGV-Funktionstasten.vi"("Aktion"=Funktionstasten-Aktion."Lesen") -> ("Busy"=w936:bool, "Betriebsart"=w940:T22)  [unwired: 7 in, 6 out]
      n472 = Equal?(x=w940, y=Betriebsart."Remote" ("Betriebsart")) -> (x = y?=w937:bool)
      n473 = case shown="True" w937 {
        tunnel: w941 -> [_ w949]
        tunnel: w933 -> [w944 w948]
        tunnel: [w943 w947] -> w934
        tunnel: w936 -> [_ w946]
        frame False {
          n474 = call "Zustandsfehlerinformation.vi"("Aktionen"=Aktionen_Zustandsfehlerinformation."Offline", "String"=w944) -> ("String"=w943:string)  [unwired: 9 in]
        }
        frame True {
          n475 = case shown="False" w946 {
            tunnel: w949 -> [w952 _]
            tunnel: w948 -> [w951 w966]
            tunnel: [w950 w965] -> w947
            frame False {
              n476 = case shown="\"K0\"" w952 {
                tunnel: w951 -> [w954 w961]
                tunnel: [w953 w960] -> w950
                frame "Standard", Default {
                  n477 = call "Zustandsfehlerinformation.vi"("Aktionen"=Aktionen_Zustandsfehlerinformation."Syntax Error", "String"=w954) -> ("String"=w953:string)  [unwired: 9 in]
                }
                frame "K0" {
                  n478 = call "FGV Automatic start.vi"("Aktion"=Aktion_FGV_Automatic_start."Seite merken") -> ("error out"=w957:errorcluster)  [unwired: 12 in, 2 out]
                  n479 = flat-sequence {
                    tunnel: w957 -> [w964]
                    tunnel: [w964] -> w956
                    frame #0 {
                      n480 = call "Bildwechsel.vi"("nächstes Bild"=Bild-Auswahl."EPA Dichtheitstest") -> ()  [unwired: 9 in, 2 out]
                    }
                  }
                  n481 = call "Zustandsfehlerinformation.vi"("Aktionen"=Aktionen_Zustandsfehlerinformation."OK", "String"=w961) -> ("String"=w960:string)  [unwired: 9 in]
                  n482 = call "FGV Automatic start.vi"("error in (no error)"=w956, "Aktion"=Aktion_FGV_Automatic_start."Test starten aktiv") -> ()  [unwired: 11 in, 3 out]
                }
              }
            }
            frame True {
              n483 = call "Zustandsfehlerinformation.vi"("Aktionen"=Aktionen_Zustandsfehlerinformation."Busy", "String"=w966) -> ("String"=w965:string)  [unwired: 9 in]
            }
          }
        }
      }
    }
    frame "SLEC" {
      n484 = call "FGV-Funktionstasten.vi"("Aktion"=Funktionstasten-Aktion."Lesen") -> ("ausgewählte Funktion"=w968:T12, "Betriebsart"=w973:T22)  [unwired: 7 in, 6 out]
      n485 = Equal?(x=w973, y=Betriebsart."Remote" ("Betriebsart")) -> (x = y?=w974:bool)
      n486 = case shown="True" w974 {
        tunnel: w970 -> [w976 w982]
        tunnel: [w975 w981] -> w969
        tunnel: w968 -> [_ w980]
        frame False {
          n487 = call "Zustandsfehlerinformation.vi"("Aktionen"=Aktionen_Zustandsfehlerinformation."Offline", "String"=w976) -> ("String"=w975:string)  [unwired: 9 in]
        }
        frame True {
          n488 = Equal?(x=w980, y=Zustaende."Standby") -> (x = y?=w978:bool)
          n489 = case shown="True" w978 {
            tunnel: w982 -> [w985 w987]
            tunnel: [w984 w986] -> w981
            frame False {
              n490 = call "Zustandsfehlerinformation.vi"("Aktionen"=Aktionen_Zustandsfehlerinformation."Datenfehler", "String"=w985) -> ("String"=w984:string)  [unwired: 9 in]
            }
            frame True {
              n491 = flat-sequence {
                frame #0 {
                  n492 = call "FGV Erweiterte Konfig.vi"("Aktion"=FGV_PID_Aktionen."Dichtheitstest", "Dichtheitstest?"=TRUE) -> ()  [unwired: 5 in, 5 out]
                }
                frame #1 {
                  n493 = vi-ref "Erweiterte Konfig.lvlib:Dichtheitstest.vi"() -> (w991:refnum<vi>)
                  n494 = call "VI Pop Up.vi"("VI Referenz"=w991) -> ()  [unwired: 11 in]
                }
              }
              n495 = call "Zustandsfehlerinformation.vi"("Aktionen"=Aktionen_Zustandsfehlerinformation."OK", "String"=w987) -> ("String"=w986:string)  [unwired: 9 in]
            }
          }
        }
      }
    }
    frame "SLES" {
      n496 = call "FGV-Funktionstasten.vi"("Aktion"=Funktionstasten-Aktion."Lesen") -> ("Betriebsart"=w997:T22)  [unwired: 7 in, 7 out]
      n497 = Equal?(x=w997, y=Betriebsart."Remote" ("Betriebsart")) -> (x = y?=w998:bool)
      n498 = case shown="True" w998 {
        tunnel: w994 -> [w1000 w1033]
        tunnel: [w999 w1032] -> w993
        tunnel: w992 -> [_ w1031]
        frame False {
          n499 = call "Zustandsfehlerinformation.vi"("Aktionen"=Aktionen_Zustandsfehlerinformation."Offline", "String"=w1000) -> ("String"=w999:string)  [unwired: 9 in]
        }
        frame True {
          n500 = Index Array(array=w1031, index #1=2 ("Index"), index #2=3 ("Index"), index #3=4 ("Index")) -> (element #1=w1005:string, element #2=w1006:string, element #3=w1007:string)
          n501 = Empty String/Path?(string/path=w1005) -> (empty?=w1010:bool)
          n502 = Empty String/Path?(string/path=w1006) -> (empty?=w1009:bool)
          n503 = Empty String/Path?(string/path=w1007) -> (empty?=w1008:bool)
          n504 = Decimal String To Number(string=w1005) -> (number=w1027:i32)  [unwired: 2 in, 1 out]
          n505 = Decimal String To Number(string=w1006) -> (number=w1023:i32)  [unwired: 2 in, 1 out]
          n506 = Decimal String To Number(string=w1007) -> (number=w1018:i32)  [unwired: 2 in, 1 out]
          n507 = Not(x=w1010) -> (.not. x?=w1004:bool)
          n508 = Not(x=w1009) -> (.not. x?=w1003:bool)
          n509 = Not(x=w1008) -> (.not. x?=w1002:bool)
          n510 = In Range and Coerce(upper limit=101 ("Obergrenze"), x=w1027, lower limit=1 ("Untergrenze")) -> (coerced(x)=w1013:i32, In Range?=w1015:bool)
          n511 = In Range and Coerce(upper limit=101 ("Obergrenze"), x=w1023, lower limit=1 ("Untergrenze")) -> (coerced(x)=w1012:i32, In Range?=w1016:bool)
          n512 = In Range and Coerce(upper limit=3 ("Obergrenze"), x=w1018, lower limit=0 ("Untergrenze")) -> (coerced(x)=w1011:i32, In Range?=w1017:bool)
          n513 = Compound Arithmetic op=AND(w1015, w1016, w1017, w1004, w1003, w1002) -> (w1014:bool)
          n514 = case shown="True" w1014 {
            tunnel: [Aktionen_Zustandsfehlerinformation."Datenfehler" ("Aktionen") Aktionen_Zustandsfehlerinformation."OK" ("Aktionen")] -> w1026
            tunnel: w1013 -> [_ w1037]
            tunnel: w1012 -> [_ w1036]
            tunnel: w1011 -> [_ w1035]
            frame False {
            }
            frame True {
              n515 = call "FGV Erweiterte Konfig.vi"("Aktion"=FGV_PID_Aktionen."Lesen") -> ("Sonstige"=w1040:T39)  [unwired: 5 in, 5 out]
              n516 = Bundle By Name(cluster=w1040, "Dichtheitstest Zeit"=w1037, "Dichtheitstest Abfall"=w1036, "Dichtheitstest Umfang"=w1035) -> (w1041:T39)
              n517 = call "FGV Erweiterte Konfig.vi"("Aktion"=FGV_PID_Aktionen."Schreiben Sonstige", "Sonstige"=w1041) -> ()  [unwired: 4 in, 6 out]
            }
          }
          n518 = call "Zustandsfehlerinformation.vi"("Aktionen"=w1026, "String"=w1033) -> ("String"=w1032:string)  [unwired: 9 in]
        }
      }
    }
    frame "SLNB" {
      n519 = call "FGV-Funktionstasten.vi"("Aktion"=Funktionstasten-Aktion."Lesen") -> ("Betriebsart"=w1048:T22)  [unwired: 7 in, 7 out]
      n520 = Equal?(x=w1048, y=Betriebsart."Remote" ("Betriebsart")) -> (x = y?=w1049:bool)
      n521 = case shown="True" w1049 {
        tunnel: w1045 -> [w1051 w1066]
        tunnel: [w1050 w1065] -> w1044
        tunnel: w1043 -> [_ w1064]
        frame False {
          n522 = call "Zustandsfehlerinformation.vi"("Aktionen"=Aktionen_Zustandsfehlerinformation."Offline", "String"=w1051) -> ("String"=w1050:string)  [unwired: 9 in]
        }
        frame True {
          # "0 oder 1"
          n523 = Index Array(array=w1064, index=2 ("Index")) -> (element=w1055:string)
          n524 = Decimal String To Number(string=w1055) -> (number=w1060:i32)  [unwired: 2 in, 1 out]
          n525 = Empty String/Path?(string/path=w1055) -> (empty?=w1054:bool)
          n526 = In Range and Coerce(upper limit=2 ("Obergrenze"), x=w1060, lower limit=0 ("Untergrenze")) -> (coerced(x)=w1056:i32, In Range?=w1058:bool)
          n527 = Not(x=w1054) -> (.not. x?=w1053:bool)
          n528 = And(x=w1058, y=w1053) -> (x .and. y?=w1057:bool)
          n529 = case shown="True" w1057 {
            tunnel: [Aktionen_Zustandsfehlerinformation."Datenfehler" ("Aktionen") Aktionen_Zustandsfehlerinformation."OK" ("Aktionen")] -> w1059
            tunnel: w1056 -> [_ w1068]
            frame False {
            }
            frame True {
              n530 = call "FGV Erweiterte Konfig.vi"("Aktion"=FGV_PID_Aktionen."Lesen") -> ("Sonstige"=w1071:T39)  [unwired: 5 in, 5 out]
              n531 = Bundle By Name(cluster=w1071, "Befüllung aktiv"=w1068) -> (w1072:T39)
              n532 = call "FGV Erweiterte Konfig.vi"("Aktion"=FGV_PID_Aktionen."Schreiben Sonstige", "Sonstige"=w1072) -> ()  [unwired: 4 in, 6 out]
            }
          }
          n533 = call "Zustandsfehlerinformation.vi"("Aktionen"=w1059, "String"=w1066) -> ("String"=w1065:string)  [unwired: 9 in]
        }
      }
    }
    frame "SMAN" {
      n534 = call "FGV-Funktionstasten.vi"("Aktion"=Funktionstasten-Aktion."Lesen") -> ("Betriebsart"=w1079:T22)  [unwired: 7 in, 7 out]
      n535 = Equal?(x=w1079, y=Betriebsart."Remote" ("Betriebsart")) -> (x = y?=w1076:bool)
      n536 = case shown="True" w1076 {
        tunnel: w1075 -> [w1082 w1085]
        tunnel: [w1080 w1084] -> w1074
        frame False {
          n537 = call "Zustandsfehlerinformation.vi"("Aktionen"=Aktionen_Zustandsfehlerinformation."Offline", "String"=w1082) -> ("String"=w1080:string)  [unwired: 9 in]
        }
        frame True {
          n538 = call "Zustandsfehlerinformation.vi"("Aktionen"=Aktionen_Zustandsfehlerinformation."OK", "String"=w1085) -> ("String"=w1084:string)  [unwired: 9 in]
          n539 = call "FGV-Funktionstasten.vi"("Aktion"=Funktionstasten-Aktion."Manuell") -> ()  [unwired: 7 in, 8 out]
        }
      }
    }
    frame "SMGA" {
      n540 = call "Setze Zustand.vi"("AK Befehl"=w1089, "Zustand"=Zustaende."Messen") -> ("Antwort String"=w1088:string)  [unwired: 8 in, 1 out]
    }
    frame "SNGA" {
      n541 = Index Array(array=w1097, index=2 ("Index")) -> (element=w1095:string)
      n542 = Decimal String To Number(string=w1095) -> (number=w1094:i32)  [unwired: 2 in, 1 out]
      n543 = Divide(x=w1094, y=10) -> (x/y=w1092:dbl)
      n544 = To Single Precision Float(number=w1092) -> (single precision float=w1090:sgl)
      n545 = call "Setze Zustand.vi"("Zeit"=w1090, "AK Befehl"=w1099, "Zustand"=Zustaende."0-Gas") -> ("Antwort String"=w1098:string)  [unwired: 7 in, 1 out]
    }
    frame "SNGF" {
      n546 = call "Setze Zustand.vi"("Befehl nicht vorhanden!"=TRUE, "AK Befehl"=w1103, "Zustand"=Zustaende."Standby") -> ("Antwort String"=w1102:string)  [unwired: 7 in, 1 out]
    }
    frame "SNOS" {
      n547 = call "FGV-Funktionstasten.vi"("Aktion"=Funktionstasten-Aktion."Lesen") -> ("Betriebsart"=w1109:T22)  [unwired: 7 in, 7 out]
      n548 = Equal?(x=w1109, y=Betriebsart."Remote" ("Betriebsart")) -> (x = y?=w1110:bool)
      n549 = case shown="True" w1110 {
        tunnel: w1106 -> [w1112 w1124]
        tunnel: [w1111 w1123] -> w1105
        tunnel: w1104 -> [_ w1122]
        frame False {
          n550 = call "Zustandsfehlerinformation.vi"("Aktionen"=Aktionen_Zustandsfehlerinformation."Offline", "String"=w1112) -> ("String"=w1111:string)  [unwired: 9 in]
        }
        frame True {
          n551 = Index Array(array=w1122, index=2 ("Index")) -> (element=w1120:string)
          n552 = Decimal String To Number(string=w1120) -> (number=w1117:i32)  [unwired: 2 in, 1 out]
          n553 = In Range and Coerce(upper limit=101 ("Obergrenze"), x=w1117, lower limit=1 ("Untergrenze")) -> (coerced(x)=w1116:i32, In Range?=w1115:bool)
          n554 = case shown="True" w1115 {
            tunnel: w1116 -> [_ w1126]
            tunnel: [Aktionen_Zustandsfehlerinformation."Datenfehler" ("Aktionen") Aktionen_Zustandsfehlerinformation."OK" ("Aktionen")] -> w1114
            frame False {
            }
            frame True {
              n555 = flat-sequence {
                tunnel: w1126 -> [w1128]
                frame #0 {
                  n556 = call "FGV FT-IR Parameter.vi"("NoOfScan neu"=w1128, "Aktion"=FGV_FT-IR_Aktionen."NOS setzen") -> ("NoOfScan"=w1129:u32)  [unwired: 10 in, 7 out]
                  n557 = call "TOOLweb SET ftirScans.vi"("ftirScans"=w1129) -> ()  [unwired: 2 in, 5 out]
                }
                frame #1 {
                  n558 = call "Queue LogFile.vi"() -> ("error out"=w1134:errorcluster, "Queue (Ausgang)"=w1133:refnum<queue>)  [unwired: 6 in]
                  n559 = call "FGV Messdaten.vi"("Aktionen"=Aktionen_FGV_Messdaten."löschen") -> ()  [unwired: 6 in, 9 out]
                  n560 = Flush Queue(queue=w1133, error in (no error)=w1134) -> (error out=w1131:errorcluster)  [unwired: 2 out]
                  n561 = call <vilib>:"Clear Errors.vi"("error in (no error)"=w1131) -> ()  [unwired: 5 in, 2 out]
                }
              }
            }
          }
          n562 = call "Zustandsfehlerinformation.vi"("Aktionen"=w1114, "String"=w1124) -> ("String"=w1123:string)  [unwired: 9 in]
        }
      }
    }
    frame "SPAU" {
      n563 = call "Setze Zustand.vi"("AK Befehl"=w1137, "Zustand"=Zustaende."Pause") -> ("Antwort String"=w1136:string)  [unwired: 8 in, 1 out]
    }
    frame "SRCP" {
      n564 = call "FGV System.vi"("Aktionen"=Aktioen_FGV_System."lesen") -> ("Optionen"=w1139:T37)  [unwired: 12 in, 6 out]
      n565 = Unbundle By Name(w1139) -> ("AK Rezeptwechsel gleich wie MKS"=w1138:bool)
      n566 = Index Array(array=w1145, index=1 ("Index")) -> (element=w1141:string)
      n567 = case shown="False" w1138 {
        tunnel: w1145 -> [w1152 w1194]
        tunnel: w1144 -> [w1151 w1182]
        tunnel: [w1150 w1183] -> w1143
        tunnel: w1141 -> [w1149 _]
        frame False {
          n568 = Equal?(x=w1149, y="K0") -> (x = y?=w1147:bool)
          n569 = case shown="True" w1147 {
            tunnel: w1152 -> [_ w1157]
            tunnel: [Aktionen_Zustandsfehlerinformation."Syntax Error" ("Aktionen") w1154] -> w1146
            frame False {
              # "Befehlskomando NICHT KORREKT!"
            }
            frame True {
              n570 = Delete From Array(array=w1157, length=2 ("Länge"), index=0 ("Index")) -> (array with subset deleted=w1156:string[])  [unwired: 1 out]
              n571 = Empty Array?(array=w1156) -> (empty?=w1155:bool)
              n572 = case shown="False" w1155 {
                tunnel: w1156 -> [w1161 _]
                tunnel: [w1162 Aktionen_Zustandsfehlerinformation."Datenfehler" ("Aktionen")] -> w1154
                frame False {
                  n573 = Index Array(array=w1161) -> (element=w1160:string)  [unwired: 1 in]
                  n574 = case shown="\"0\", Standard" w1160 {
                    tunnel: [Aktionen_Zustandsfehlerinformation."OK" ("Aktionen") Aktionen_Zustandsfehlerinformation."Syntax Error" ("Aktionen") Aktionen_Zustandsfehlerinformation."OK" ("Aktionen") Aktionen_Zustandsfehlerinformation."OK" ("Aktionen")] -> w1162
                    frame "CNG" {
                      n575 = call "FGV Rezepte wechseln.vi"("AK/man"=AK-manuell."CNG", "Aktion"=Aktion_FGV_Rezepte_wechseln."AK/Man") -> ("error out"=w1165:errorcluster)  [unwired: 7 in, 6 out]
                      n576 = flat-sequence {
                        tunnel: w1165 -> [_]
                        frame #0 {
                          n577 = vi-ref "FT-IR.lvlib:TOOLweb Interface.lvlib:TOOLweb Rezept wechseln.vi"() -> (w1167:refnum<vi>)
                          n578 = call "VI Pop Up.vi"("VI Referenz"=w1167) -> ()  [unwired: 11 in]
                        }
                      }
                    }
                    frame "0", Default {
                    }
                    frame "DIESEL" {
                      n579 = call "FGV Rezepte wechseln.vi"("AK/man"=AK-manuell."Diesel", "Aktion"=Aktion_FGV_Rezepte_wechseln."AK/Man") -> ("error out"=w1171:errorcluster)  [unwired: 7 in, 6 out]
                      n580 = flat-sequence {
                        tunnel: w1171 -> [_]
                        frame #0 {
                          n581 = vi-ref "FT-IR.lvlib:TOOLweb Interface.lvlib:TOOLweb Rezept wechseln.vi"() -> (w1173:refnum<vi>)
                          n582 = call "VI Pop Up.vi"("VI Referenz"=w1173) -> ()  [unwired: 11 in]
                        }
                      }
                    }
                    frame "GASOLINE" {
                      n583 = call "FGV Rezepte wechseln.vi"("AK/man"=AK-manuell."Gasoline", "Aktion"=Aktion_FGV_Rezepte_wechseln."AK/Man") -> ("error out"=w1176:errorcluster)  [unwired: 7 in, 6 out]
                      n584 = flat-sequence {
                        tunnel: w1176 -> [_]
                        frame #0 {
                          n585 = vi-ref "FT-IR.lvlib:TOOLweb Interface.lvlib:TOOLweb Rezept wechseln.vi"() -> (w1178:refnum<vi>)
                          n586 = call "VI Pop Up.vi"("VI Referenz"=w1178) -> ()  [unwired: 11 in]
                        }
                      }
                    }
                  }
                }
                frame True {
                  # "Fehler mit den Einstell Kommandos"
                }
              }
            }
          }
          n587 = call "Zustandsfehlerinformation.vi"("Aktionen"=w1146, "String"=w1151) -> ("String"=w1150:string)  [unwired: 9 in]
        }
        frame True {
          n588 = Array Subset(array=w1194, index=1 ("Index")) -> (w1192:string[])  [unwired: 1 in]
          n589 = Array Size(array=w1192) -> (size(s)=w1191:i32)
          n590 = for {
            tunnel: w1192 -> [w1210] mode=indexing
            tunnel: [w1209] -> w1190 mode=indexing
            tunnel: w1191 -> [w1208]
            i -> [w1206]
            n591 = Decrement(x=w1208) -> (x-1=w1207:i32)
            n592 = Equal?(x=w1207, y=w1206) -> (x = y?=w1205:bool)
            n593 = case shown="False" w1205 {
              tunnel: w1210 -> [w1213 w1214]
              tunnel: [w1211 w1214] -> w1209
              frame False {
                n594 = call <vilib>:"Space Constant.vi"() -> ("String"=w1212:string)
                n595 = Concatenate Strings(w1213, w1212) -> (w1211:string)
              }
              frame True {
              }
            }
          }
          n596 = call "FGV Rezepte wechseln.vi"("AK/man"=AK-manuell."manuell", "Aktion"=Aktion_FGV_Rezepte_wechseln."AK/Man") -> ("Rezepte"=w1187:string[])  [unwired: 7 in, 6 out]
          n597 = Concatenate Strings(w1190) -> (w1186:string)
          n598 = for {
            tunnel: w1187 -> [w1204] mode=indexing
            tunnel: w1186 -> [w1203]
            tunnel: [w1201] -> w1185 mode=indexing if=w1202
            i -> [w1201]
            n599 = Equal?(x=w1204, y=w1203) -> (x = y?=w1202:bool)
          }
          n600 = Empty Array?(array=w1185) -> (empty?=w1181:bool)
          n601 = Index Array(array=w1185) -> (element=w1180:i32)  [unwired: 1 in]
          n602 = case shown="False" w1181 {
            tunnel: [Aktionen_Zustandsfehlerinformation."OK" ("Aktionen") Aktionen_Zustandsfehlerinformation."Syntax Error" ("Aktionen")] -> w1184
            tunnel: w1180 -> [w1196 _]
            frame False {
              n603 = call "FGV Rezepte wechseln.vi"("Rezeptindex"=w1196, "Aktion"=Aktion_FGV_Rezepte_wechseln."Rezeptindex") -> ("error out"=w1195:errorcluster)  [unwired: 7 in, 6 out]
              n604 = flat-sequence {
                tunnel: w1195 -> [_]
                frame #0 {
                  n605 = vi-ref "FT-IR.lvlib:TOOLweb Interface.lvlib:TOOLweb Rezept wechseln.vi"() -> (w1199:refnum<vi>)
                  n606 = call "VI Pop Up.vi"("VI Referenz"=w1199) -> ()  [unwired: 11 in]
                }
              }
            }
            frame True {
            }
          }
          n607 = call "Zustandsfehlerinformation.vi"("Aktionen"=w1184, "String"=w1182) -> ("String"=w1183:string)  [unwired: 9 in]
        }
      }
    }
    frame "SREM" {
      n608 = call "Zustandsfehlerinformation.vi"("Aktionen"=Aktionen_Zustandsfehlerinformation."OK", "String"=w1216) -> ("String"=w1215:string)  [unwired: 9 in]
      n609 = call "FGV-Funktionstasten.vi"("Aktion"=Funktionstasten-Aktion."Remote") -> ()  [unwired: 7 in, 8 out]
    }
    frame "SRUC" {
      n610 = Index Array(array=w1220, index=2 ("Index")) -> (element=w1224:string)
      n611 = Decimal String To Number(string=w1224) -> (number=w1223:i32)  [unwired: 2 in, 1 out]
      n612 = Divide(x=w1223, y=10) -> (x/y=w1221:dbl)
      n613 = To Single Precision Float(number=w1221) -> (single precision float=w1219:sgl)
      n614 = call "Setze Zustand.vi"("Zeit"=w1219, "AK Befehl"=w1228, "Zustand"=Zustaende."Spülen Filter") -> ("Antwort String"=w1227:string)  [unwired: 7 in, 1 out]
    }
    frame "SSBE" {
      n615 = Index Array(array=w1230, index=1 ("Index")) -> (element=w1232:string)
      n616 = call "FGV-Funktionstasten.vi"("Aktion"=Funktionstasten-Aktion."Lesen") -> ("Betriebsart"=w1238:T22)  [unwired: 7 in, 7 out]
      n617 = Equal?(x=w1238, y=Betriebsart."Remote" ("Betriebsart")) -> (x = y?=w1239:bool)
      n618 = Equal?(x=w1232, y="K0") -> (x = y?=w1229:bool)
      n619 = case shown="True" w1229 {
        tunnel: w1239 -> [_ w1246]
        tunnel: w1235 -> [w1241 w1245]
        tunnel: [w1240 w1244] -> w1234
        tunnel: w1230 -> [_ w1243]
        frame False {
          n620 = call "Zustandsfehlerinformation.vi"("Aktionen"=Aktionen_Zustandsfehlerinformation."OK", "String"=w1241) -> ("String"=w1240:string)  [unwired: 9 in]
        }
        frame True {
          n621 = case shown="True" w1246 {
            tunnel: w1245 -> [w1248 w1255]
            tunnel: [w1247 w1254] -> w1244
            tunnel: w1243 -> [_ w1253]
            frame False {
              n622 = call "Zustandsfehlerinformation.vi"("Aktionen"=Aktionen_Zustandsfehlerinformation."Offline", "String"=w1248) -> ("String"=w1247:string)  [unwired: 9 in]
            }
            frame True {
              n623 = Index Array(array=w1253, index=2 ("Index")) -> (element=w1250:string)
              n624 = Empty String/Path?(string/path=w1250) -> (empty?=w1251:bool)
              n625 = case shown="False" w1251 {
                tunnel: w1255 -> [w1257 w1262]
                tunnel: [w1256 w1261] -> w1254
                tunnel: w1250 -> [_ w1260]
                frame True {
                  n626 = call "Zustandsfehlerinformation.vi"("Aktionen"=Aktionen_Zustandsfehlerinformation."Datenfehler", "String"=w1257) -> ("String"=w1256:string)  [unwired: 9 in]
                }
                frame False {
                  n627 = call "Zustandsfehlerinformation.vi"("Aktionen"=Aktionen_Zustandsfehlerinformation."OK", "String"=w1262) -> ("String"=w1261:string)  [unwired: 9 in]
                  n628 = call "TOOLweb SET LABFILE BaseName.vi"("BaseName"=w1260) -> ("error out"=w1259:errorcluster)  [unwired: 2 in, 4 out]
                  n629 = call <vilib>:"Clear Errors.vi"("error in (no error)"=w1259) -> ()  [unwired: 5 in, 2 out]
                }
              }
            }
          }
        }
      }
    }
    frame "SSLO" {
      n630 = Index Array(array=w1265, index=1 ("Index")) -> (element=w1267:string)
      n631 = call "FGV-Funktionstasten.vi"("Aktion"=Funktionstasten-Aktion."Lesen") -> ("Betriebsart"=w1273:T22)  [unwired: 7 in, 7 out]
      n632 = Equal?(x=w1273, y=Betriebsart."Remote" ("Betriebsart")) -> (x = y?=w1274:bool)
      n633 = Equal?(x=w1267, y="K0") -> (x = y?=w1264:bool)
      n634 = case shown="True" w1264 {
        tunnel: w1274 -> [_ w1281]
        tunnel: w1270 -> [w1276 w1280]
        tunnel: [w1275 w1279] -> w1269
        tunnel: w1265 -> [_ w1278]
        frame False {
          n635 = call "Zustandsfehlerinformation.vi"("Aktionen"=Aktionen_Zustandsfehlerinformation."Syntax Error", "String"=w1276) -> ("String"=w1275:string)  [unwired: 9 in]
        }
        frame True {
          n636 = case shown="True" w1281 {
            tunnel: w1280 -> [w1283 w1288]
            tunnel: [w1282 w1287] -> w1279
            tunnel: w1278 -> [_ w1294]
            frame False {
              n637 = call "Zustandsfehlerinformation.vi"("Aktionen"=Aktionen_Zustandsfehlerinformation."Offline", "String"=w1283) -> ("String"=w1282:string)  [unwired: 9 in]
            }
            frame True {
              n638 = Index Array(array=w1294, index #1=2 ("Index"), index #2=3 ("Index")) -> (element #1=w1286:string, element #2=w1291:string)
              n639 = Empty String/Path?(string/path=w1286) -> (empty?=w1285:bool)
              n640 = Decimal String To Number(string=w1286) -> (number=w1289:i32)  [unwired: 2 in, 1 out]
              n641 = Decimal String To Number(string=w1291) -> (number=w1290:i32)  [unwired: 2 in, 1 out]
              n642 = case shown="False" w1285 {
                tunnel: w1290 -> [w1298 _]
                tunnel: w1289 -> [w1297 _]
                tunnel: w1288 -> [w1296 w1313]
                tunnel: [w1295 w1312] -> w1287
                frame False {
                  n643 = case shown="2, Standard" w1297 {
                    tunnel: w1298 -> [_ w1307 _]
                    tunnel: w1296 -> [w1300 w1305 w1309]
                    tunnel: [w1299 w1304 w1308] -> w1295
                    frame 0 {
                      n644 = disable-structure shown="Deaktiviert" {
                        frame Disabled {
                          n645 = call "FGV Spektren automatisch aufzeichnen.vi"("Aktion"=Aktion_FGV_Spektren_automatisch_aufzeichnen."reset") -> ()  [unwired: 14 in, 1 out]
                        }
                        frame Enabled {
                        }
                      }
                      n646 = call "Zustandsfehlerinformation.vi"("Aktionen"=Aktionen_Zustandsfehlerinformation."OK", "String"=w1300) -> ("String"=w1299:string)  [unwired: 9 in]
                    }
                    frame 1 {
                      n647 = call "Zustandsfehlerinformation.vi"("Aktionen"=Aktionen_Zustandsfehlerinformation."OK", "String"=w1305) -> ("String"=w1304:string)  [unwired: 9 in]
                      n648 = call "FGV Spektren automatisch aufzeichnen.vi"("Zeit"=w1307, "Aktion"=Aktion_FGV_Spektren_automatisch_aufzeichnen."set") -> ()  [unwired: 13 in, 1 out]
                    }
                    frame 2, Default {
                      n649 = call "Zustandsfehlerinformation.vi"("Aktionen"=Aktionen_Zustandsfehlerinformation."Syntax Error", "String"=w1309) -> ("String"=w1308:string)  [unwired: 9 in]
                    }
                  }
                }
                frame True {
                  n650 = call "Zustandsfehlerinformation.vi"("Aktionen"=Aktionen_Zustandsfehlerinformation."Syntax Error", "String"=w1313) -> ("String"=w1312:string)  [unwired: 9 in]
                }
              }
            }
          }
        }
      }
    }
    frame "SSNR" {
      n651 = Index Array(array=w1315, index=1 ("Index")) -> (element=w1317:string)
      n652 = call "FGV-Funktionstasten.vi"("Aktion"=Funktionstasten-Aktion."Lesen") -> ("Betriebsart"=w1323:T22)  [unwired: 7 in, 7 out]
      n653 = Equal?(x=w1323, y=Betriebsart."Remote" ("Betriebsart")) -> (x = y?=w1324:bool)
      n654 = Equal?(x=w1317, y="K0") -> (x = y?=w1314:bool)
      n655 = case shown="True" w1314 {
        tunnel: w1324 -> [_ w1331]
        tunnel: w1320 -> [w1326 w1330]
        tunnel: [w1325 w1329] -> w1319
        tunnel: w1315 -> [_ w1328]
        frame False {
          n656 = call "Zustandsfehlerinformation.vi"("Aktionen"=Aktionen_Zustandsfehlerinformation."OK", "String"=w1326) -> ("String"=w1325:string)  [unwired: 9 in]
        }
        frame True {
          n657 = case shown="True" w1331 {
            tunnel: w1330 -> [w1333 w1341]
            tunnel: [w1332 w1340] -> w1329
            tunnel: w1328 -> [_ w1339]
            frame False {
              n658 = call "Zustandsfehlerinformation.vi"("Aktionen"=Aktionen_Zustandsfehlerinformation."Offline", "String"=w1333) -> ("String"=w1332:string)  [unwired: 9 in]
            }
            frame True {
              n659 = Index Array(array=w1339, index=2 ("Index")) -> (element=w1337:string)
              n660 = Decimal String To Number(string=w1337) -> (number=w1336:i32)  [unwired: 2 in, 1 out]
              n661 = call "TOOLweb SET LABINDEX.vi"("SPEC#:"=w1336) -> ("error out"=w1335:errorcluster)  [unwired: 4 in, 2 out]
              n662 = call "Zustandsfehlerinformation.vi"("Aktionen"=Aktionen_Zustandsfehlerinformation."OK", "String"=w1341) -> ("String"=w1340:string)  [unwired: 9 in]
              n663 = call <vilib>:"Clear Errors.vi"("error in (no error)"=w1335) -> ()  [unwired: 5 in, 2 out]
            }
          }
        }
      }
    }
    frame "SSPL" {
      n664 = Index Array(array=w1344, index=2 ("Index")) -> (element=w1348:string)
      n665 = Decimal String To Number(string=w1348) -> (number=w1347:i32)  [unwired: 2 in, 1 out]
      n666 = Divide(x=w1347, y=10) -> (x/y=w1345:dbl)
      n667 = To Single Precision Float(number=w1345) -> (single precision float=w1343:sgl)
      n668 = call "Setze Zustand.vi"("Zeit"=w1343, "AK Befehl"=w1352, "Zustand"=Zustaende."Spülen Leitung") -> ("Antwort String"=w1351:string)  [unwired: 7 in, 1 out]
    }
    frame "SSPR" {
      n669 = call "Setze Zustand.vi"("Befehl nicht vorhanden!"=TRUE, "AK Befehl"=w1356, "Zustand"=Zustaende."Standby") -> ("Antwort String"=w1355:string)  [unwired: 7 in, 1 out]
    }
    frame "STBY" {
      n670 = call "Setze Zustand.vi"("AK Befehl"=w1359, "Zustand"=Zustaende."Standby") -> ("Antwort String"=w1358:string)  [unwired: 8 in, 1 out]
    }
    frame "STRG" {
      n671 = call "FGV-Funktionstasten.vi"("Aktion"=Funktionstasten-Aktion."Lesen") -> ("Betriebsart"=w1365:T22)  [unwired: 7 in, 7 out]
      n672 = Equal?(x=w1365, y=Betriebsart."Remote" ("Betriebsart")) -> (x = y?=w1366:bool)
      n673 = case shown="False" w1366 {
        tunnel: w1362 -> [w1368 w1375]
        tunnel: [w1367 w1374] -> w1361
        tunnel: w1360 -> [_ w1373]
        frame False {
          n674 = call "Zustandsfehlerinformation.vi"("Aktionen"=Aktionen_Zustandsfehlerinformation."Offline", "String"=w1368) -> ("String"=w1367:string)  [unwired: 9 in]
        }
        frame True {
          n675 = Index Array(array=w1373, index=2 ("Index")) -> (element=w1371:string)
          n676 = Empty String/Path?(string/path=w1371) -> (empty?=w1370:bool)
          n677 = case shown="False" w1370 {
            tunnel: w1375 -> [w1382 w1395]
            tunnel: [w1381 w1394] -> w1374
            tunnel: w1371 -> [w1380 _]
            frame False {
              n678 = Decimal String To Number(string=w1380) -> (number=w1377:i32)  [unwired: 2 in, 1 out]
              n679 = In Range and Coerce(upper limit=2 ("Obergrenze"), x=w1377, lower limit=0 ("Untergrenze")) -> (In Range?=w1376:bool)  [unwired: 1 out]
              n680 = case shown="False" w1376 {
                tunnel: w1382 -> [w1384 w1392]
                tunnel: [w1383 w1391] -> w1381
                tunnel: w1377 -> [_ w1386]
                frame False {
                  n681 = call "Zustandsfehlerinformation.vi"("Aktionen"=Aktionen_Zustandsfehlerinformation."Datenfehler", "String"=w1384) -> ("String"=w1383:string)  [unwired: 9 in]
                }
                frame True {
                  # "Wenn informationen da sind, dann übergeben!"
                  n682 = call "FGV Trigger.vi"("Aktion"=Aktionen_Trigger."lesen") -> ("Triggerereignis neu"=w1388:T47)  [unwired: 7 in, 3 out]
                  n683 = Bundle By Name(cluster=w1388, "Trigger verwenden"=w1386) -> (w1387:T47)
                  n684 = call "Zustandsfehlerinformation.vi"("Aktionen"=Aktionen_Zustandsfehlerinformation."OK", "String"=w1392) -> ("String"=w1391:string)  [unwired: 9 in]
                  n685 = call "FGV Trigger.vi"("Aktion"=Aktionen_Trigger."ALLE schreiben", "Triggerereignis"=w1387) -> ()  [unwired: 6 in, 4 out]
                }
              }
            }
            frame True {
              # "Wenn nur STRG dann Trigger setzen!!!"
              n686 = call "FGV Trigger.vi"("Aktion"=Aktionen_Trigger."Trigger prüfen", "Trigger setzen"=TRUE) -> ()  [unwired: 6 in, 4 out]
              n687 = call "Zustandsfehlerinformation.vi"("Aktionen"=Aktionen_Zustandsfehlerinformation."OK", "String"=w1395) -> ("String"=w1394:string)  [unwired: 9 in]
            }
          }
        }
      }
    }
  }
  "String für schreiben" <- w5
